vi "3Danalysis240909 cropcalibration with real-time waveforms.vi"() -> ()   [LabVIEW 2024]
uses:
  <vilib>/Utility/file.llb/Read Delimited Spreadsheet (DBL).vi
  <vilib>/Utility/file.llb/Read Delimited Spreadsheet (string).vi
  Global variables/filepath global variable.vi
  Global variables/global for picoscope.vi
  <vilib>/Utility/file.llb/Write Delimited Spreadsheet (DBL).vi
  <vilib>/Utility/file.llb/Write Delimited Spreadsheet (I64).vi
panel:
  in  "round-trip":bool
  in  "fit results":bool
  in  "correction":T1={"vibration removal"=FALSE, "x correct fast/slow"=TRUE, "y correct fast/slow"=TRUE, "z correct fast/slow"=TRUE}
  out "max ch2":u16
  out "max ch1":u16=17224
  out "volume rate [Hz]":dbl=450.6612227351971
  in  "batch":bool
  out "config":bool
  in  "save config":bool
  in  "init frame ofst ch1":dbl
  out "path":path
  out "z ofst":dbl
  in  "auto z adjust":T2={"margin"=100.0, "auto z adj"=FALSE, "average"=10, "use given ofst"=FALSE, "given ofst"=0}
  in  "save file":enum16{"3DU16", "avi", "avia.tif", "none"}(ring)=enum."avia.tif"
  in  "init volume":i64 min=-1 max=9995
  out "Numeric":i32
  out "x-y":dbl=0.003430600045248866
  in  "vol ofst for filesave":i32
  out "x-y 2":dbl=154.19183529983275
  out "x-y 3":dbl=0.0007527999114245176
  in  "save all":bool=TRUE
  out "Array":u16[](array[numeric])=[1044]
  out "Array 2":u16[](array[numeric])
  out "Waveform Graph 8":u16[](graph)=[1044]
  out "Waveform Graph 7":u16[](graph)
  out "Waveform Graph 3":u16[](graph)
  in  "# of vols to save":u32=9 max=9996
  in  "init frame ofst ch2":dbl
  in  "calib using picoscope":bool
  out "error out 2":errorcluster
  out "cal":bool=TRUE
  out "static cropcalib ch2":dbl[][][](array[numeric])
  out "static cropcalib ch1":dbl[][][](array[numeric])=[[[-0.0012324508841086526, -13.277704725109043, 0.9825265622945943, 0.013882930010711092], [-9.275883597421803, 40.97187002025559, 0.26309128953548033, 0.01695088157165565]], [[-0.0037120993202699767, 133.57085155510373, 0.31941814051590384, 0.021131841125054136], [-9.390393874751965, 181.5531741318331, -0.10717785095280981, 0.018933425267278654]], [[0.0019777746813413695, 278.58470887012226, 0.12331601194921626, 0.017358112403776993], [-9.300617403370904, 321.6599217146224, -0.408166255458373, 0.007869360209962234]], [[0.003878363727042984, 422.57664944690487, 0.012423017399425418, 0.008011499786472465], [-9.810808384161477, 461.18609374492786, -0.022657621769615152, 0.006436963821634987]], [[-0.005737681625292825, 565.5516858154322, 0.2650733563737, 0.011263202764196095], [-9.832152645016635, 600.6762263679414, -0.30527039372187453, 0.010318730252671056]], [[8.042249450854295e-07, 707.5829139794733, -0.1207414064195435, 0.0023412830187913803], [-9.87910924649735, 739.8216036823347, 0.005640673976347694, -0.0005605768217188439]], [[-0.01334711027106098, 848.5600859130332, 0.12422403037488547, 0.002919715456556465], [-9.442660667127637, 878.9222143445218, 0.2884952700379346, -0.0006542554942195691]], [[0.0, 990.0108512212238, 0.0, 0.0], [-9.33364564551871, 1018.373465441547, 0.10671859828055268, -0.0003399303862730855]], [[0.0, 1130.6258231987185, 0.0, 0.0], [-9.580976920588036, 1157.4289207081854, -0.046484964058340905, -0.0023746044096836305]], [[0.19067519003123512, 1271.6329414805725, 0.28218230543582085, -0.004007953579247134], [-9.478759959162836, 1296.7982093928567, 0.06815273675590765, -0.005249059904662809]], [[0.002910935849795122, 1411.5924221171872, 0.23076489126866379, -0.0035025104155532653], [-9.327754021590689, 1436.6481286976045, -0.15077568684339113, 0.002054927352480896]], [[0.0045119752683153375, 1551.6884161105997, 0.9967475870149168, 0.005783955565654333], [-9.342246137492738, 1576.5099590441323, -0.036967108722480435, -0.0015882138039450067]], [[0.0012251998944222717, 1691.7091671736623, 0.8828208157286062, 0.004890461811581429], [-8.991691053184148, 1717.2464623070055, 0.42353732985143466, 0.008074427179974693]], [[0.04480350158940928, 1831.6789885716557, 0.2702553130960064, 0.008058123936945851], [-9.520266895758336, 1858.7924624587888, 0.13922336686163864, 0.012889168242776554]], [[0.006579691004563718, 1972.5865362020297, -0.31771324719759314, 0.011874761201387155], [-9.693713496805085, 2000.6691119313275, 0.28434979045685604, 0.006521998044205342]], [[-0.00011619691447528437, 2113.575841906626, 0.027477117752841233, 0.008658919164037509], [-8.4059148140794, 2144.426688166775, -0.0013392330480600891, 0.0034757601889036393]]]
  out "ref image":u16[][](graph)
  out "merged 2":picture
  in  "first calib?":bool
  in  "calib folder":path=path "E:/20241013-235052zebrafish-cropbulkcalib"
  in  "man x correct":dbl[](array[numeric])=[0.0, 0.0, 0.0, 0.0, 0.0, 0.0, 0.0, 0.0, 0.0, 0.0, 0.0, 0.0, 0.0, 0.0, 0.0, 0.0] format="%_3g"
  out "xcutcalib":bool
  in  "save xcutcalib":bool
  out "Waveform Graph 6":dbl[][](graph)
  in  "add xcutcalib":bool
  out "Waveform Graph 5":dbl[][](graph)=[[71.24917145755833, 2.611229946524065], [52.12883880825057, 96.52276455026455], [38.370065789473685, 37.02559300873908], [109.29258898776419, 117.5164798671648], [109.03552721356218, 113.07896244046542], [107.5345264511574, 111.91266505636071], [101.79099323375462, 108.80995217599235], [81.80626577898215, 91.38536842105262], [76.35199183363878, 81.89281794462502], [72.85646288715512, 77.08998393172541], [70.33839267741641, 73.63359060670481], [68.91633042357225, 71.23733432369326], [68.61642295097899, 70.59161782206286], [67.06026334942868, 69.3341155147388], [67.74688487608418, 68.88457267871622], [67.23388367805843, 67.52512049939843]]
  out "Waveform Graph 4":dbl[][](graph)=[[70.75082854244167, 12.808059587471355, 2.629934210526315, 14.534830367074527, 16.427308035479975, 17.7857922739422, 22.1671837099451, 9.975237111191262, 9.040092700463049, 10.394476704747461, 12.436049890733301, 13.007639351673383, 13.537171153329393, 13.652122809925942, 13.660225864725732, 13.787552156319304], [2.611229946524065, 2.787949735449729, 2.7521847690387027, 14.601328352013269, 18.22516127087478, 18.055853462157813, 21.7295600191296, 12.989368421052625, 8.892359420239849, 10.20478995530609, 12.280460403088203, 13.044423160691835, 13.582757039632213, 13.732063344670266, 13.630206965107035, 13.843818558527587]]
  out "calib errors":dbl[][](graph)=[[71.24917145755833, 52.12883880825057, 38.370065789473685, 109.29258898776419, 109.03552721356218, 107.5345264511574, 101.79099323375462, 81.80626577898215, 76.35199183363878, 72.85646288715512, 70.33839267741641, 68.91633042357225, 68.61642295097899, 67.06026334942868, 67.74688487608418, 67.23388367805843], [2.611229946524065, 96.52276455026455, 37.02559300873908, 117.5164798671648, 113.07896244046542, 111.91266505636071, 108.80995217599235, 91.38536842105262, 81.89281794462502, 77.08998393172541, 73.63359060670481, 71.23733432369326, 70.59161782206286, 69.3341155147388, 68.88457267871622, 67.52512049939843]]
  out "Waveform Graph 2":u64[][](graph)
  out "mag corr ch2":dbl=0.9999999999999987
  out "size(s) 2":i32[](array[numeric])=[344, 346]
  out "#ofvoxels":i32[](array[numeric])=[2, 144, 2304]
  in  "y shift comp ch2":dbl=2.0 format="%_4g"
  out "# of slices per frame":dbl=16.0
  out "coeffs ch2":T3={"coeffs for r adjust"=[519.0152004188965, 310.5655915232708, 70.01299823861439, 7.02374490371761, 0.263935632321602], "coeffs for x pos adjust"=[1129.1985384616178, -0.06820417207386949, 3.261911031170097e-08, -3.700712469960341e-12, -2.2526696193466402e-15, 2.275859361243603e-19, 4.209771129915532e-23, -5.09041527821271e-27, -4.152675622145259e-31, 5.315442386029638e-35, 2.2654166541347624e-39, -2.8567558128164638e-43, -6.398399651393965e-48, 7.62901113711002e-52, 7.223314072712311e-57, -8.008405878791859e-61], "coeffs for intensity adjust"=[0.058988135271943375, -6.250993723417386e-05, 8.465587569932774e-07, -2.944632303001578e-09, 4.603084712096755e-12, -3.778602476142126e-15, 1.6979803184001706e-18, -3.9600508630542766e-22, 3.7530066428820694e-26]}
  out "coeffs ch1":T3={"coeffs for r adjust"=[17.10761405696684, 7.84114849852129, 1.7677363155338985, 0.2069198771701287, 0.00932990152601304], "coeffs for x pos adjust"=[1127.3789093477487, -0.06827960368149495, 3.2476822001437325e-08, 1.2710261197144785e-13, -1.3608202177260485e-15, 1.4043859987815547e-21, 2.104622239338711e-23, 2.30596280455575e-28, -2.3225210012230083e-31, -9.089899485608927e-36, 2.1092005655095755e-39, 9.893885524186623e-44, -1.2826034157079897e-47, -4.393969803780215e-52, 4.214036083794186e-56, 6.97605374735289e-61, -5.591200085114606e-65], "coeffs for intensity adjust"=[0.25889415470638116, -0.00016368169857389878, 1.1910443462708163e-08, -7.647385084110969e-10, 1.8842781690841883e-12, -1.906465046959414e-15, 9.982378310740631e-19, -2.6840743111736396e-22, 2.938746954924419e-26]}
  out "img scan voltage":dbl[][](array[numeric])
  out "img scan tangent":dbl[][](array[numeric])
  out "calib index":i32
  out "Waveform Graph":u32[][](graph)=[[15301, 15180, 15264, 15156, 15317, 15620, 15556, 15291, 15455, 15405, 15401, 15373, 15584, 15573, 15767, 15492, 15691, 15604, 15561, 15794, 15664, 15376, 15642, 15407, 15469, 15364, 15405, 15434, 15394, 15413, 15350, 15460, 15316, 15440, 15429, 15553, 15564, 15422, 15390, 15723, 15577, 15625, 15805, 15738, 15559, 15673, 15778, 15951, 15719, 15813, 15643, 15950, 15843, 15867, 15752, 15687, 15565, 15831, 15737, 15690, 15741, 15588, 15471, 15668, 15745, 15718, 15687, 15627, 15417, 15716, 15742, 15760, 15744, 15903, 15757, 15817, 15715, 15772, 15822, 15917, 15764, 15955, 15688, 15823, 15723, 15617, 15641, 15498, 15509, 15540, 15467, 15681, 15463, 15503, 15416, 15393, 15441, 15439, 15466, 15298, 15311, 15441, 15260, 15298, 15258, 15267, 15341, 15224, 15222, 15120, 15226, 15313, 15275, 15176, 15268, 15210, 15155, 15201, 15095, 15249, 15176, 15248, 15220, 15296, 15148, 15124, 15152, 15276, 15240, 15128, 15162, 15171, 15217, 15209, 15238, 15355, 15305, 15141, 15199, 15275, 15223, 15324, 15184, 15222, 15158, 15279, 15288, 15313, 15254, 15159, 15370, 15393, 15448, 15274, 15475, 15438, 15469, 15554, 15779, 15661, 15709, 15811, 15752, 15747, 15674, 15677, 15732, 15441, 15664, 15538, 15479, 15524, 15353, 15443, 15486, 15434, 15412, 15413, 15332, 15417, 15385, 15511, 15304, 15327, 15381, 15325, 15492, 15474, 15428, 15381, 15710, 15723, 15643, 15578, 15595, 15577, 15710, 15546, 15584, 15590, 15497, 15653, 15634, 15476, 15548, 15538, 15617, 15466, 15546, 15575, 15482, 15436, 15510, 15547, 15364, 15570, 15524, 15525, 15401, 15598, 15591, 15501, 15572, 15609, 15540, 15693, 15490, 15453, 15613, 15544, 15603, 15536, 15393, 15609, 15422, 15500, 15552, 15330, 15306, 15418, 15271, 15374, 15347, 15270, 15334, 15281, 15261, 15290, 15296, 15137, 15348, 15212, 15159, 15360, 15150, 15233, 15106, 15189, 15153, 15232, 15155, 15364, 15279, 15248, 15187, 15153, 15122, 15164, 15379, 15274, 15347, 15249, 15096, 15359, 15362, 15224, 15313, 15428, 15264, 15307, 15212, 15090, 15264, 15277, 15291, 15138, 15253, 15329, 15351, 15295, 15246, 15360, 15238, 15463, 15316, 15448, 15364, 15595, 15507, 15632, 15755, 16022, 16075, 16206, 16022, 16142, 16221, 16087, 15909, 15837, 15636, 15936, 15910, 15764, 15799, 15649, 15868, 15776, 15651, 15764, 15618, 15379, 15599, 15447, 15560, 15468, 15370, 15563, 15391, 15358, 15343, 15440, 15501, 15404, 15597, 15488, 15308, 15516, 15654, 15472, 15411, 15486, 15716, 15512, 15710, 15658, 15524, 15441, 15730, 15407, 15472, 15352, 15539, 15410, 15505, 15504, 15409, 15402, 15634, 15370, 15422, 15453, 15528, 15406, 15400, 15524, 15386, 15511, 15444, 15512, 15377, 15500, 15715, 15412, 15544, 15388, 15328, 15393, 15459, 15265, 15314, 15280, 15236, 15370, 15422, 15418, 15205, 15193, 15347, 15173, 15370, 15242, 15228, 15060, 15265, 15166, 15148, 15284, 15223, 15229, 15300, 15278, 15142, 15058, 15158, 15119, 15289, 15124, 15233, 15118, 15208, 15111, 15234, 15133, 15042, 15094, 15042, 15032, 15002, 15002, 14881, 14742, 14852, 14737, 14936, 14673, 14649, 14760, 14733, 14748, 14659, 14623, 14658, 14696, 14688, 14762, 14665, 14769, 14866, 14937, 15108, 14998, 15277, 15463, 15587, 15444, 15777, 15716, 15491, 15710, 15500, 15671, 15793, 15788, 15636, 15796, 15739, 15537, 15236, 15566, 15438, 15293, 15155, 15182, 15237, 15280, 15128, 15231, 14931, 15277, 14907, 14833, 14939, 14989, 14857, 14833, 14881, 14717, 14877, 14883, 14851, 14867, 14821, 14647, 14814, 14897, 14835, 14793, 14950, 14956, 14795, 14876, 14850, 14888, 14865, 14696, 14836, 14783, 14891, 14790, 14911, 14817, 14898, 14793, 14971, 14870, 14925, 14735, 14810, 14636, 14845, 14818, 14698, 14750, 14783, 14724, 14762, 14697, 14790, 14881, 14914, 14826, 14649, 14710, 14946, 14827, 14735, 14720, 14626, 14787, 14673, 14606, 14648, 14823, 14654, 14549, 14721, 14744, 14830, 14769, 14608, 14568, 14724, 14723, 14668, 14814, 14601, 14710, 14865, 14640, 14657, 14722, 14646, 14625, 14607, 14694, 14631, 14864, 14665, 14746, 14790, 14679, 14656, 14511, 14679, 14547, 14610, 14816, 14836, 14622, 14726, 15028, 14747, 14699, 14809, 14849, 14934, 14798, 15011, 14970, 14942, 14926, 15361, 15383, 15318, 15654, 15568, 15877, 15922, 16129, 16325, 16195, 16142, 16324, 15970, 16153, 16258, 16122, 16121, 15864, 15996, 15776, 15984, 15895, 15770, 15641, 15841, 15542, 15614, 15569, 15408, 15432, 15397, 15399, 15281, 15335, 15037, 15085, 14974, 15158, 15012, 14836, 15038, 14777, 14954, 14924, 14903, 14761, 14934, 14849, 14847, 14636, 14963, 14896, 14905, 14930, 15016, 14904, 14889, 14977, 14884, 14887, 14727, 14785, 14783, 14768, 14720, 14690, 14917, 14744, 14840, 14804, 14766, 14829, 14834, 14711, 14745, 14869, 14833, 14779, 14742, 14837, 14866, 14951, 14722, 14784, 14727, 14825, 14674, 14801, 14805, 14658, 14887, 14875, 14775, 14606, 14616, 14529, 14680, 14740, 14578, 14672, 14813, 14756, 14670, 14693, 14612, 14793, 14597, 14734, 14679, 14724, 14685, 14677, 14654, 14655, 14678, 14675, 14513, 14571, 14668, 14665, 14616, 14624, 14663, 14614, 14754, 14637, 14634, 14619, 14753, 14686, 14505, 14700, 14550, 14684, 14589, 14762, 14776, 14836, 14635, 14801, 15007, 15117, 15100, 15439, 15491, 15771, 15906, 16022, 16368, 16512, 16330, 16351, 16557, 16465, 16406, 16234, 16591, 16446, 16480, 16250, 16315, 16147, 16060, 16079, 16094, 15904, 15863, 15932, 15882, 15891, 15683, 15596, 15649, 15525, 15478, 15666, 15460, 15409, 15276, 15227, 15141, 15230, 15059, 15197, 14980, 14852, 14745, 14895, 14902, 14975, 14783, 14747, 14806, 14615, 14725, 14654, 14869, 14645, 14679, 14727, 14569, 14636, 14908, 14606, 14674, 14774, 14843, 14803, 14841, 14843, 14818, 14781, 14918, 14820, 14756, 14862, 14753, 14709, 14728, 14766, 14850, 14664, 14686, 14748, 14838, 14594, 14634, 14706, 14604, 14633, 14584, 14693, 14670, 14469, 14631, 14633, 14634, 14639, 14533, 14704, 14649, 14757, 14567, 14679, 14508, 14521, 14695, 14630, 14850, 14637, 14665, 14690, 14741, 14705, 14606, 14787, 14585, 14653, 14552, 14709, 14690, 14607, 14611, 14761, 14773, 14690, 14538, 14702, 14738, 14767, 14710, 14460, 14620, 14837, 14753, 14661, 14781, 14701, 14799, 14908, 14827, 15123, 15229, 15246, 15510, 15604, 15760, 16237, 16402, 16499, 16640, 16630, 16865, 16713, 16772, 16986, 17048, 16820, 17014, 17012, 16803, 16863, 16755, 16959, 16780, 16746, 16827, 16793, 16578, 16902, 16565, 16658, 16675, 16497, 16458, 16430, 16427, 16376, 16348, 16316, 16314, 16299, 16308, 16615, 16241, 16331, 16279, 16335, 16241, 15910, 15826, 15634, 15615, 15284, 15254, 15096, 14971, 14700, 14734, 14773, 14798, 14644, 14652, 14671, 14674, 14664, 14511, 14692, 14763, 14704, 14759, 14553, 14655, 14653, 14709, 14624, 14626, 14798, 14717, 14682, 14534, 14682, 14583, 14548, 14461, 14605, 14458, 14579, 14654, 14660, 14631, 14606, 14737, 14701, 14810, 14597, 14712, 14469, 14742, 14784, 14763, 14537, 14784, 14711, 14880, 14778, 14801, 14789, 14826, 14816, 14795, 14786, 15015, 14997, 14956, 15024, 14709, 14923, 14843, 15055, 15216, 14971, 15234, 15172, 14933, 15048, 15215, 14970, 15048, 14963, 15170, 15194, 15187, 14911, 14855, 15080, 15189, 15258, 15303, 15139, 15331, 15551, 15836, 15861, 15969, 16312, 16430, 16568, 16676, 17392, 17468, 17768, 17693, 17963, 18003, 17922, 18241, 18356, 18506, 18505, 18693, 18834, 18522, 18645, 18971, 18831, 19145, 19262, 19202, 19282, 19163, 19920, 19966, 20063, 20348, 20393, 20656, 20340, 21145, 21549, 21592, 22895, 23897, 24817, 26484, 27677, 28989, 30335, 31522, 32712, 33150, 33951, 34337, 33384, 33011, 31426, 29622, 27294, 25484, 23051, 20348, 19043, 17525, 16719, 16071, 15893, 15557, 15642, 15478, 15709, 15737, 15436, 15783, 15635, 15433, 15632, 15632, 15509, 15537, 15450, 15605, 15399, 15681, 15592, 15674, 15625, 15525, 15509, 15757, 15625, 15765, 15896, 16007, 15916, 15913, 15957, 15909, 16022, 15915, 16044, 15928, 16205, 16212, 15998, 16200, 15978, 16027, 16055, 16251, 16221, 15986, 15900, 16181, 16011, 16126, 16144, 16104, 15950, 16110, 16250, 16178, 15817, 15999, 15876, 15970, 15988, 16103, 16080, 16090, 16142, 16097, 15951, 16043, 16001, 16185, 16033, 16197, 16194, 16187, 16293, 16448, 16389, 16439, 16771, 16725, 17242, 17347, 17859, 18357, 18497, 19124, 18931, 19384, 19557, 19681, 20120, 20401, 20902, 20890, 21244, 21383, 21631, 21445, 21859, 21581, 22396, 22624, 22629, 22872, 23615, 23902, 24218, 24837, 25984, 27149, 28740, 29966, 31555, 33231, 34755, 35668, 37514, 41116, 44002, 48952, 53923, 60849, 67906, 75888, 84944, 92910, 100381, 107495, 114716, 119015, 121334, 123649, 124437, 120797, 114049, 105794, 96821, 84687, 70486, 58082, 44862, 35256, 27393, 22565, 19113, 17558, 16721, 16534, 16333, 16339, 16347, 16226, 16349, 16177, 16227, 16152, 16088, 16127, 16170, 16022, 16206, 16060, 15819, 15950, 16096, 15893, 16030, 15980, 15961, 15897, 15997, 16092, 15901, 16154, 16074, 16032, 16079, 15908, 15981, 15858, 15948, 15991, 15950, 15907, 15791, 15741, 15870, 15941, 15946, 15786, 15735, 15883, 15833, 15812, 15917, 15778, 15816, 15824, 15904, 16092, 15925, 15850, 15892, 15870, 16134, 16127, 15951, 15940, 16044, 15942, 15967, 16154, 16178, 16250, 16305, 16374, 16485, 16677, 17020, 17399, 17653, 18134, 18430, 18725, 19268, 19703, 20036, 20607, 20881, 21617, 21808, 22208, 22703, 23272, 23742, 24224, 25206, 25741, 26436, 26115, 26837, 27022, 27879, 28914, 29039, 30172, 31220, 32066, 33038, 33999, 35051, 35854, 37878, 40694, 44209, 48835, 53423, 59090, 66638, 73627, 84244, 93544, 107457, 122595, 140161, 158551, 176805, 195989, 216903, 237255, 253503, 268650, 279752, 288924, 294235, 297628, 296038, 287332, 278665, 263556, 243244, 221305, 195837, 166539, 136516, 105426, 75906, 53503, 39346, 29244, 22700, 19333, 18204, 17399, 17089, 17127, 16970, 16678, 16734, 16750, 16657, 16567, 16785, 16628, 16332, 16398, 16470, 16429, 16394, 16557, 16197, 16424, 16217, 16243, 16481, 16269, 16480, 16195, 16094, 16229, 16129, 16155, 16125, 16097, 16103, 15991, 16154, 15764, 16125, 16167, 16082, 16010, 15905, 16131, 15931, 16049, 16092, 16023, 16103, 16091, 16012, 16082, 15955, 16083, 16025, 16045, 15977, 16060, 16144, 16213, 16027, 16082, 16235, 16311, 16377, 16503, 16775, 16862, 17475, 17701, 18469, 18731, 19442, 19969, 20370, 21112, 21671, 22136, 23022, 23572, 24091, 24722, 25933, 26396, 26817, 27431, 28425, 29086, 29942, 30624, 31583, 33102, 34332, 35298, 36413, 37376, 38747, 39967, 43311, 47174, 49971, 54701, 57287, 59902, 63295, 66811, 71971, 78251, 87577, 99880, 113736, 131859, 153016, 178039, 206189, 239140, 268322, 301593, 333225, 367689, 398869, 428520, 451155, 475148, 489399, 497230, 503148, 496024, 486052, 473743, 459727, 440198, 423502, 401541, 378537, 350159, 317117, 283508, 249811, 212312, 172174, 130532, 93652, 63983, 45225, 34266, 26456, 22357, 19836, 18750, 18252, 17894, 17777, 17481, 17485, 17554, 17437, 17303, 17283, 17111, 17217, 17206, 17221, 17107, 17105, 16961, 16998, 16806, 16832, 16863, 16808, 16803, 16745, 16679, 16747, 16551, 16469, 16574, 16435, 16529, 16401, 16521, 16386, 16392, 16523, 16342, 16525, 16259, 16297, 16355, 16263, 16338, 16314, 16273, 16224, 16130, 16484, 16470, 16374, 16335, 16439, 16365, 16735, 16643, 16905, 17006, 17275, 17985, 18159, 19047, 19437, 20108, 20875, 21610, 22120, 22948, 24140, 24131, 25489, 26193, 26968, 28297, 29738, 30483, 31666, 32227, 33636, 34398, 34059, 35223, 36490, 36884, 38504, 40271, 41945, 44509, 47280, 48477, 51090, 54262, 56936, 61006, 66133, 71868, 79670, 88305, 99993, 111659, 128041, 143678, 164564, 188426, 212219, 243102, 279213, 317533, 361157, 407173, 451353, 496387, 540920, 589454, 628126, 669232, 700813, 723519, 745001, 753018, 752391, 740749, 723123, 691046, 658326, 620040, 572513, 527741, 480657, 444358, 410016, 378605, 350538, 322320, 291428, 258834, 225020, 189363, 152976, 118813, 86963, 61562, 44560, 34493, 27353, 24224, 21579, 19913, 19389, 19236, 18812, 18744, 18724, 18475, 18422, 18363, 18216, 18115, 17977, 17841, 17896, 18034, 17844, 18199, 17500, 17515, 17515, 17496, 17497, 17255, 17290, 17574, 17424, 17177, 17375, 17090, 17144, 17219, 17022, 17080, 17145, 16820, 17223, 17039, 17189, 16899, 17020, 16870, 16910, 16866, 17041, 16979, 16909, 17002, 16944, 17150, 17566, 17899, 18236, 18515, 19087, 19838, 20625, 21161, 22236, 23021, 23997, 24730, 25887, 27082, 27799, 28365, 29108, 30249, 31803, 32735, 33182, 34289, 35800, 37800, 38796, 40330, 41050, 42229, 44197, 45186, 46340, 47995, 51153, 53820, 57457, 60830, 66370, 70884, 76806, 82883, 88504, 96097, 106036, 119146, 135853, 159213, 184956, 218869, 257150, 303167, 351380, 404496, 461094, 516175, 572027, 633124, 688319, 738230, 787014, 827991, 854865, 881463, 896306, 910597, 913862, 913067, 906683, 890807, 865170, 831071, 795584, 754028, 709973, 662118, 605784, 549409, 483865, 419856, 360697, 315672, 280400, 253947, 234130, 214854, 194686, 173041, 149605, 127645, 104234, 84306, 65189, 51366, 39446, 32019, 26412, 23264, 21272, 20159, 19385, 18610, 18414, 18093, 18490, 17971, 17983, 17783, 17851, 17674, 17628, 17318, 17252, 17442, 17439, 17331, 17261, 17127, 17244, 16886, 16953, 16784, 16641, 16852, 16628, 16669, 16711, 16434, 16638, 16463, 16581, 16567, 16486, 16240, 16433, 16524, 16551, 16194, 16391, 16314, 16489, 16680, 17180, 17175, 17711, 18422, 19049, 19979, 21200, 21935, 22972, 23556, 25590, 26261, 27006, 28339, 28906, 30104, 30911, 32480, 33461, 35388, 36464, 37352, 38800, 40399, 41320, 42713, 45053, 47280, 49848, 52384, 54499, 58600, 60782, 63994, 67586, 69716, 74103, 77534, 84424, 91208, 99851, 110435, 124005, 137527, 155612, 178442, 202188, 235450, 273699, 319248, 372231, 433490, 501830, 576537, 653111, 732092, 812185, 889041, 962405, 1033476, 1096394, 1142818, 1173475, 1192354, 1200630, 1192201, 1172933, 1139546, 1089841, 1040146, 986591, 927992, 870181, 806735, 746934, 685563, 632047, 584453, 533421, 482557, 433064, 381002, 323084, 266939, 216421, 175486, 147291, 125611, 112236, 104304, 94351, 85259, 75673, 66289, 57941, 50597, 43241, 38954, 33458, 29350, 25379, 23511, 21532, 20226, 19809, 18965, 18703, 18501, 18209, 18260, 18141, 17817, 17809, 18016, 17674, 17697, 17429, 17443, 17414, 17227, 17312, 17028, 17105, 17088, 17094, 17016, 16913, 16813, 16998, 16852, 16557, 16827, 16800, 16751, 16651, 16644, 16786, 16902, 17043, 17034, 17564, 17724, 18440, 19136, 19888, 20738, 21984, 23073, 24714, 25388, 26621, 28099, 29669, 30688, 32055, 32735, 34008, 35241, 35868, 37543, 38391, 39021, 40822, 42295, 45423, 45800, 49099, 50955, 52919, 55654, 59539, 62706, 67003, 70922, 76452, 82783, 89017, 95961, 102930, 111409, 118810, 128557, 140490, 154271, 170561, 192744, 221950, 258542, 301489, 352767, 409571, 475568, 546229, 620262, 699762, 783523, 874514, 959011, 1044943, 1120847, 1187540, 1248777, 1293721, 1333230, 1359942, 1379028, 1382262, 1379460, 1359103, 1327999, 1285059, 1231617, 1164257, 1091238, 1007154, 928419, 844405, 757878, 676229, 597066, 528033, 463441, 413333, 374781, 335717, 300607, 263367, 229745, 193155, 160808, 128937, 102926, 82811, 67352, 56486, 49754, 45587, 42542, 40256, 38294, 35989, 34950, 33131, 31780, 29795, 27955, 26516, 24316, 22921, 21806, 20404, 19737, 19399, 19001, 18452, 18706, 18467, 18304, 18158, 18056, 17919, 17801, 18174, 17694, 17760, 17705, 17767, 17437, 17521, 17338, 17410, 17443, 17280, 17343, 17149, 17543, 17318, 17788, 17827, 17840, 18200, 18793, 19208, 19827, 20694, 21466, 22573, 23700, 24945, 25659, 27197, 29110, 29533, 31317, 32834, 34114, 34715, 36219, 38039, 38475, 39989, 41731, 43043, 44588, 45833, 47268, 48769, 49436, 51832, 54445, 57775, 59840, 63742, 67764, 70830, 75375, 81209, 87777, 93275, 103706, 112868, 125799, 137302, 156220, 175226, 197889, 226567, 257984, 297377, 341021, 390206, 450937, 522808, 601241, 691414, 781338, 882139, 984069, 1085111, 1187802, 1288509, 1381524, 1463138, 1534083, 1585526, 1617605, 1633580, 1624674, 1600301, 1560683, 1505553, 1441754, 1362876, 1288571, 1214588, 1136801, 1063451, 994504, 918425, 842202, 764751, 681209, 603591, 530105, 463057, 397166, 338045, 287495, 243163, 208503, 181413, 163218, 144555, 128059, 114225, 99374, 87439, 75751, 67156, 57580, 50017, 43598, 38676, 34192, 31828, 30513, 29648, 28873, 28263, 27857, 27605, 26534, 26224, 25603, 24809, 22981, 22510, 21546, 20835, 19857, 19264, 19073, 18890, 18430, 18477, 18180, 18055, 18322, 17982, 17782, 17589, 17392, 17555, 17257, 17398, 17054, 16987, 16721, 16538, 16379, 16262, 15924, 15643, 15674, 15358, 15222, 15328, 15019, 14994, 15002, 15053, 14869, 14782, 14709, 14755, 14624, 14632, 14699, 14720, 14786, 14800, 14606, 14729, 14808, 14642, 14714, 14677, 14568, 14415, 14610, 14635, 14451, 14498, 14499, 14383, 14464, 14469, 14470, 14537, 14432, 14429, 14424, 14405]]
  in  "init vol":i32
  in  "skip":i32=30 min=1
  out "coeffs":bool
  out "error out":errorcluster
  out "config cluster":T4={"xy cut pos correct"=[[0.0, 0.0], [0.0, 0.0], [0.0, 0.0], [0.0, 0.0], [0.0, 0.0], [0.0, 0.0], [0.0, 0.0], [0.0, 0.0], [0.0, 0.0], [0.0, 0.0], [0.0, 0.0], [0.0, 0.0], [0.0, 0.0], [0.0, 0.0], [0.0, 0.0], [0.0, 0.0]], "3D reconst config"={"xyz pos"=[68, 22, 14], "color 4"={"color array"=[0, 8388736, 16711680, 16776960, 16776960, 16711680, 16448250, 16448250], "num of colors"=4, "max"=7000.900000000023, "min"=100.0}, "autogain"=TRUE, "zoom"=1.0, "slice(T)/stack(F)"=FALSE, "xy cut mag"=0.999999999999986, "xy cut ofst"=0.0, "z/xy comp"=1.0, "y shift comp"=0.0, "max plot"=TRUE, "oblique angle [deg]"=0.0, "voxel size z [um]"=2.47291183688844, "voxel size xy[um]"=0.4095, "reverse v"=FALSE, "reverse h"=TRUE, "3D reconstruction"=TRUE, "reverse z"=FALSE}, "xy cut pos"=[[0.0, 0.0], [0.0, 0.0], [0.0, 0.0], [0.0, 0.0], [0.0, 0.0], [0.0, 0.0], [0.0, 0.0], [0.0, 0.0], [0.0, 0.0], [0.0, 0.0], [0.0, 0.0], [0.0, 0.0], [0.0, 0.0], [0.0, 0.0], [0.0, 0.0], [0.0, 0.0]], "AOD scan speed ratio"=7.0, "Nx"=142.71428571, "stack method"=enum."0pad to x", "y shift"=-3}
  out "voxel number":i32[](array[numeric])=[32, 141, 143]
  in  "Zoom 2":sgl=1.9000002 format="%_3g"
  in  "Cluster 2":T5={"colors 2"=[{"color array"=[0, 16711680, 16776960, 16448250, 16776960, 16711680, 16448250, 16448250], "num of colors"=4, "max"=20300.0, "min"=100.0}, {"color array"=[0, 65280, 16711680, 16448250, 16776960, 16711680, 16448250, 16448250], "num of colors"=2, "max"=400.0, "min"=140.0}, {"color array"=[0, 16711680, 16448250, 16448250, 16776960, 16711680, 16448250, 16448250], "num of colors"=2, "max"=12500.0, "min"=0.0}, {"color array"=[0, 255, 16448250, 16448250, 16776960, 16711680, 16448250, 16448250], "num of colors"=2, "max"=1.01, "min"=0.0}, {"color array"=[0, 65280, 16448250, 16448250, 16776960, 16711680, 16448250, 16448250], "num of colors"=3, "max"=1.0, "min"=0.0}, {"color array"=[0, 255, 16448250, 16448250, 16776960, 16711680, 16448250, 16448250], "num of colors"=2, "max"=1.0099999999999991, "min"=0.0}], "on/off 2"=[TRUE, TRUE, FALSE, FALSE, FALSE, FALSE], "fast/slow"=TRUE, "on/off"=TRUE} {"colors 2"."min" step=0.01 format="%_2f"; "colors 2"."max" step=0.1 format="%_3f"}
  out "voxel size":dbl[](array[numeric])=[2.47291183688844, 0.4095, 0.4095]
  in  "stack method":T6(ring)=enum."0pad to x"
  out "# of volumes":dbl=2500.0
  out "roop time":dbl=0.7064968999984558
  in  "most recent":bool
  in  "folderpath":path=path "E:/20241013-235254zebrafish"
  out "timestamp":dbl[](array[numeric]) format="%#_12g"
  out "int frame ch2":dbl
  out "int frame ch1":dbl
  out "bytes per frame":i64=663560
  out "frames per vol":dbl=2.0
  in  "3D config":T7={"xyz pos"=[68, 22, 14], "color 4"={"color array"=[0, 8388736, 16711680, 16776960, 16776960, 16711680, 16448250, 16448250], "num of colors"=4, "max"=7000.900000000023, "min"=100.0}, "autogain"=TRUE, "zoom"=1.0, "slice(T)/stack(F)"=FALSE, "xy cut mag"=0.999999999999986, "xy cut ofst"=0.0, "z/xy comp"=1.0, "y shift comp"=0.0, "max plot"=TRUE, "oblique angle [deg]"=0.0, "voxel size z [um]"=2.47291183688844, "voxel size xy[um]"=0.4095, "reverse v"=FALSE, "reverse h"=TRUE, "3D reconstruction"=TRUE, "reverse z"=FALSE} {"oblique angle [deg]" format="%_4g"; "y shift comp" format="%_4g"; "z/xy comp" format="%_4g"; "xy cut mag" format="%_4g"; "zoom" format="%_3g"; "color 4"."min" step=0.01 format="%_2f"; "color 4"."max" step=0.1 format="%_3f"}
  in  "mag correct":dbl=0.9999999999999999 format="%_5g"
  in  "2color":bool
  out "basic info":dbl[](array[numeric])=[2.0, 16.0, 142.71428571, 7.0, 1105.2, 10.0]
  in  "page":i32
  out "# of frames":dbl=5000.0
  out "frame's init pos in x":dbl[][](array[numeric])=[[0.0, 1835.00901738322], [114.51851696314236, 1721.147101789565], [232.0020802680026, 1603.7715933557456], [348.14555636837696, 1489.3931858186936], [462.566358639522, 1375.7385908149276], [579.2325307907199, 1258.8475197694584], [693.9573343258472, 1145.2327344550233], [808.0498359122519, 1031.3113628318458], [924.0289031657775, 915.7950185906724], [1037.9895674693335, 802.6538134765885], [1151.8597552062292, 688.8875445391162], [1266.303305871278, 573.8303042476285], [1379.5189602745013, 460.50349291965074], [1492.7992407967668, 346.3820388319155], [1607.3275809299998, 231.6954939592598], [1721.0230196410016, 118.6551055908842]]
  out "time intervals":dbl[][](graph)
  in  "vol index":i64 min=-1 max=49
  in  "stop":bool
  in  "rel mag ch2":dbl=0.9999999999999988 format="%_5g"
  in  "v shift":i32=-3
  in  "h shift":i32=-9
  out "merged":picture
  out "monitor index":i32=68
  # "1ボリュームあたりのカメラフレーム数\nカメラフレームあたりのXYフレーム数\nXYフレームのＸピクセル数\nratio between AOD & img scan\ng2 period [us]\ndead time for burst [us]"
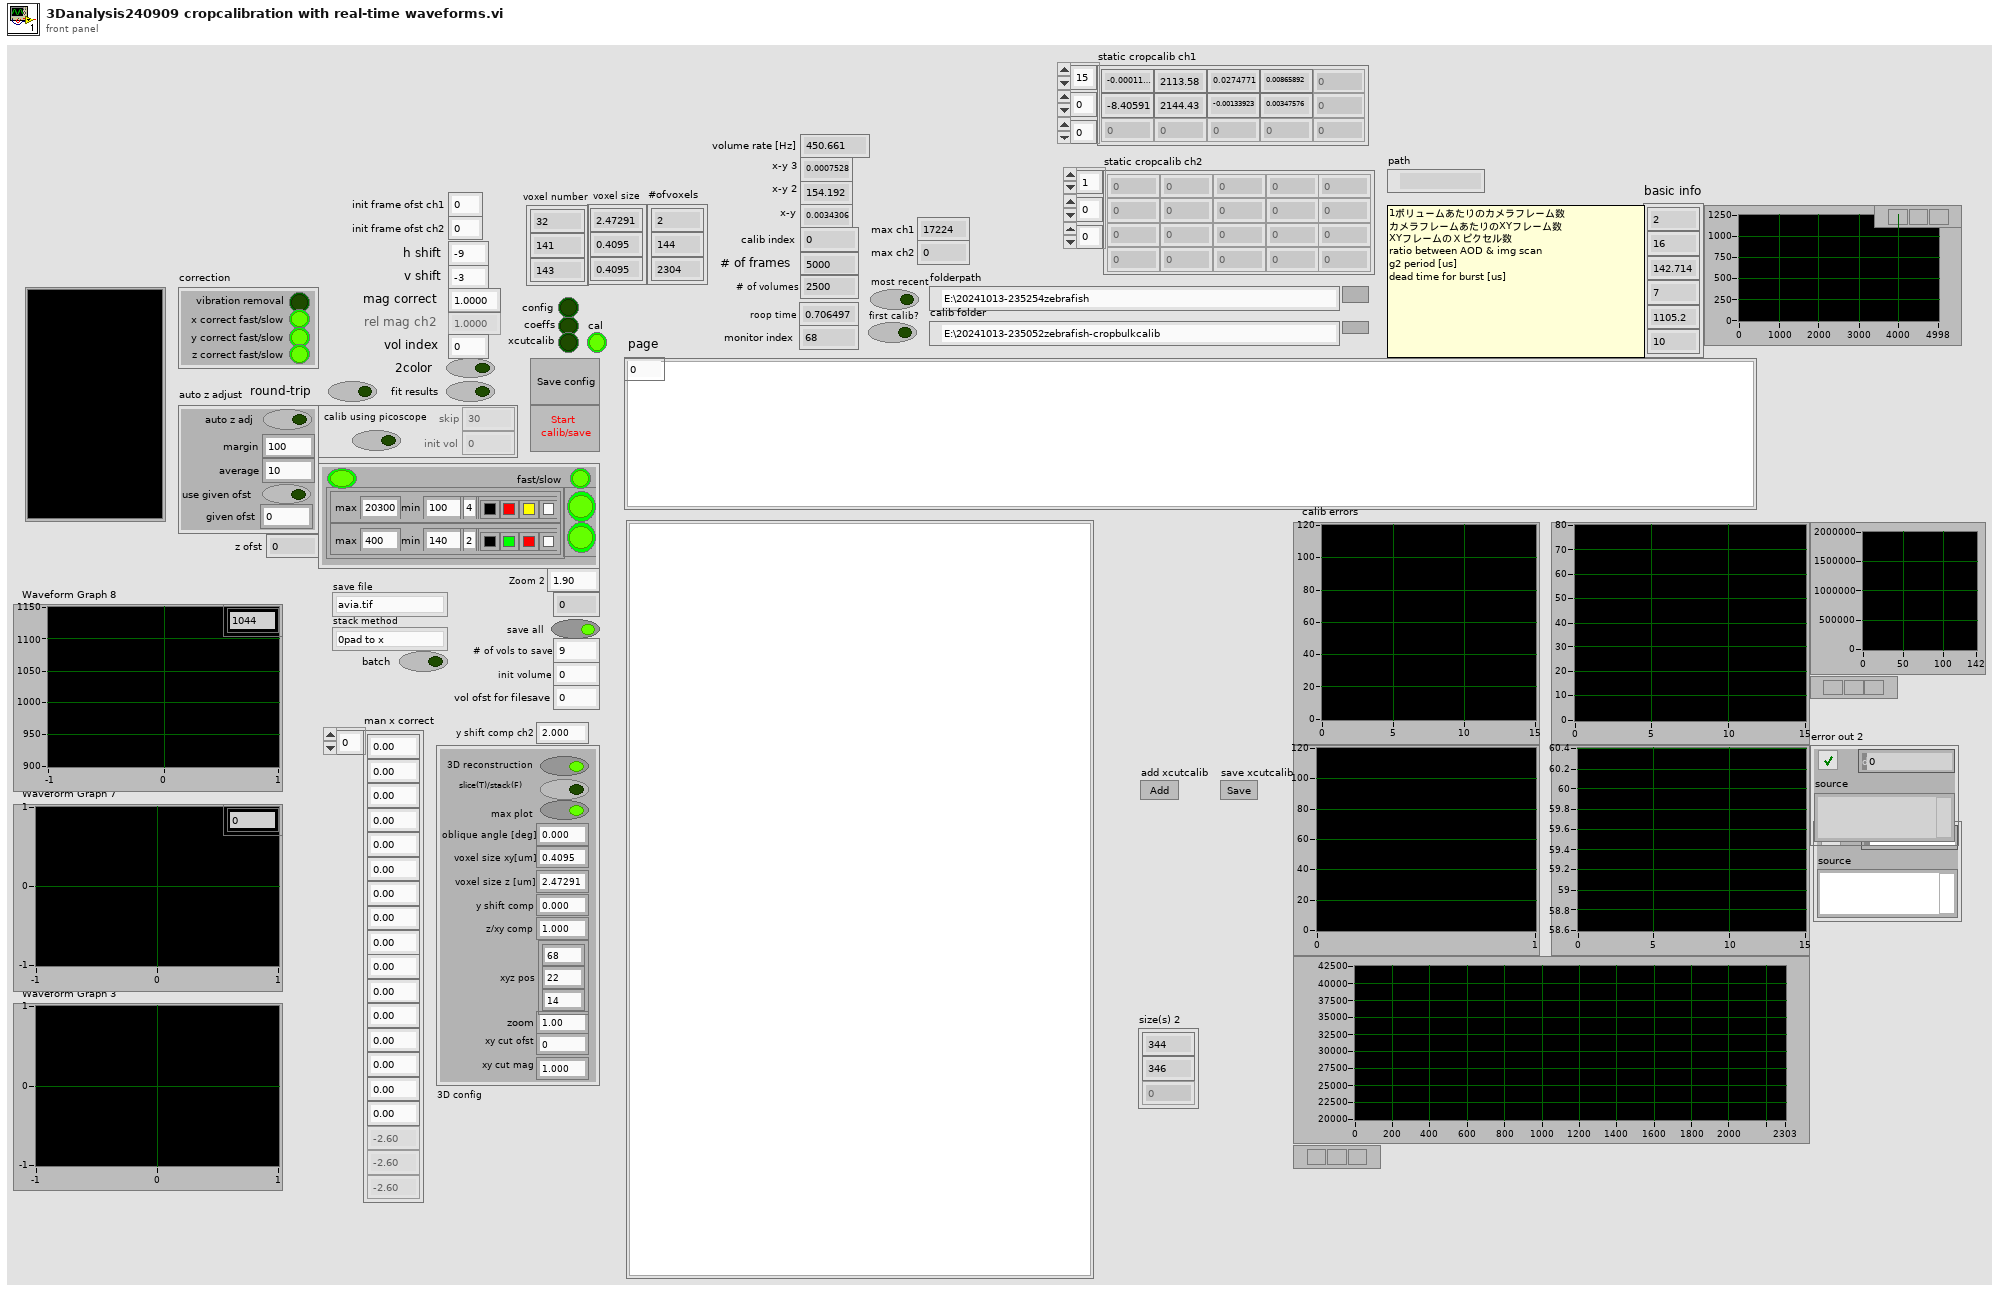
[diagram p1: front panel]
types:
  T1 = cluster{"vibration removal":bool, "x correct fast/slow":bool, "y correct fast/slow":bool, "z correct fast/slow":bool}
  T2 = cluster{"margin":dbl, "auto z adj":bool, "average":i32, "use given ofst":bool, "given ofst":i32}
  T3 = cluster{"coeffs for r adjust":dbl[], "coeffs for x pos adjust":dbl[], "coeffs for intensity adjust":dbl[]}
  T4 = cluster{"xy cut pos correct":dbl[][], "3D reconst config":cluster{"xyz pos":u16[], "color 4":cluster{"color array":u32[], "num of colors":i32, "max":dbl, "min":dbl}, "autogain":bool, "zoom":dbl, "slice(T)/stack(F)":bool, "xy cut mag":dbl, "xy cut ofst":dbl, "z/xy comp":dbl, "y shift comp":dbl, "max plot":bool, "oblique angle [deg]":dbl, "voxel size z [um]":dbl, "voxel size xy[um]":dbl, "reverse v":bool, "reverse h":bool, "3D reconstruction":bool, "reverse z":bool}, "xy cut pos":dbl[][], "AOD scan speed ratio":dbl, "Nx":dbl, "stack method":enum16{"0pad to z", "0pad to x", "0pad to x and rot"}, "y shift":i32}
  T5 = cluster{"colors 2":cluster{"color array":u32[], "num of colors":i32, "max":dbl, "min":dbl}[], "on/off 2":bool[], "fast/slow":bool, "on/off":bool}
  T6 = enum16{"0pad to z", "0pad to x", "0pad to x and rot"}
  T7 = cluster{"xyz pos":u16[], "color 4":cluster{"color array":u32[], "num of colors":i32, "max":dbl, "min":dbl}, "autogain":bool, "zoom":dbl, "slice(T)/stack(F)":bool, "xy cut mag":dbl, "xy cut ofst":dbl, "z/xy comp":dbl, "y shift comp":dbl, "max plot":bool, "oblique angle [deg]":dbl, "voxel size z [um]":dbl, "voxel size xy[um]":dbl, "reverse v":bool, "reverse h":bool, "3D reconstruction":bool, "reverse z":bool}
  T8 = cluster{"img scan pos":dbl[][], "g1 disp [um]":dbl, "z spacing [um]":dbl, "g2 disp [pixels]":dbl, "scape scan pos ":dbl[]}
  T9 = cluster{"config cluster":cluster{"xy cut pos correct":dbl[][], "3D reconst config":cluster{"xyz pos":u16[], "color 4":cluster{"color array":u32[], "num of colors":i32, "max":dbl, "min":dbl}, "autogain":bool, "zoom":dbl, "slice(T)/stack(F)":bool, "xy cut mag":dbl, "xy cut ofst":dbl, "z/xy comp":dbl, "y shift comp":dbl, "max plot":bool, "oblique angle [deg]":dbl, "voxel size z [um]":dbl, "voxel size xy[um]":dbl, "reverse v":bool, "reverse h":bool, "3D reconstruction":bool, "reverse z":bool}, "xy cut pos":dbl[][], "AOD scan speed ratio":dbl, "Nx":dbl, "stack method":enum16{"0pad to z", "0pad to x", "0pad to x and rot"}, "y shift":i32}, "optimized param":dbl[][][][][], "volume indices":i32[]}
  T10 = cluster{"coeffs":cluster{"coeffs for r adjust":dbl[], "coeffs for x pos adjust":dbl[], "coeffs for intensity adjust":dbl[]}[], "config for coeffs":cluster{"# of avg for single waveform":u16, "skip [us]":dbl, "Nzf*Nv":i32, "ofst":dbl, "# of avg for volumes":u16, "limit data length":bool, "num of frames":i32, "Nv":i32}}
  T11 = enum16{"open", "replace", "create", "open or create", "replace or create", "replace or create with confirmation"}
  T12 = cluster{"img scan tangent":dbl[][], "img scan voltage":dbl[][]}
  T13 = cluster{"# of avg for single waveform":u16, "skip [us]":dbl, "Nzf*Nv":i32, "ofst":dbl, "# of avg for volumes":u16, "limit data length":bool, "num of frames":i32, "Nv":i32}
  T14 = cluster{"coeffs for r adjust":dbl[], "coeffs for x pos adjust":dbl[], "coeffs for intensity adjust":dbl[]}[]
  T15 = enum8{"Enabled", "Disabled", "Disabled and Grayed Out"}
  T16 = typedef "IMAQ AVI2 Refnum.ctl" = refnum<k20>
  T17 = typedef "Image Type" = u32
  T18 = typedef "IMAQ Image.ctl" = refnum<image>
  T19 = cluster{"color array":u32[], "num of colors":i32, "max":dbl, "min":dbl}[]
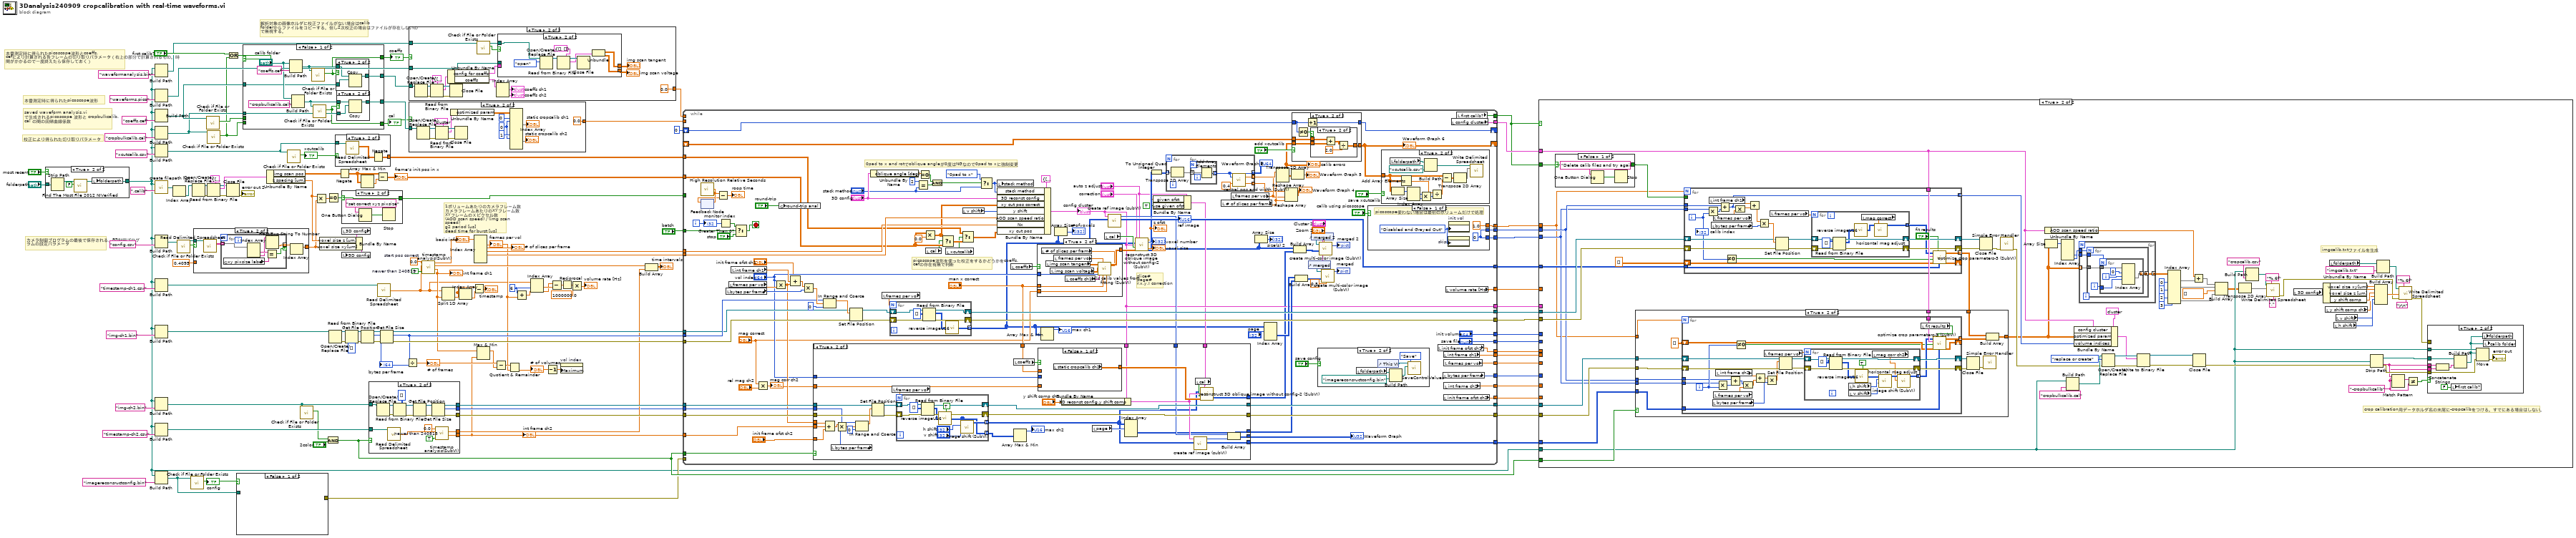
[diagram p0: block diagram]
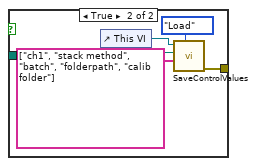
[diagram p2: hidden frame]
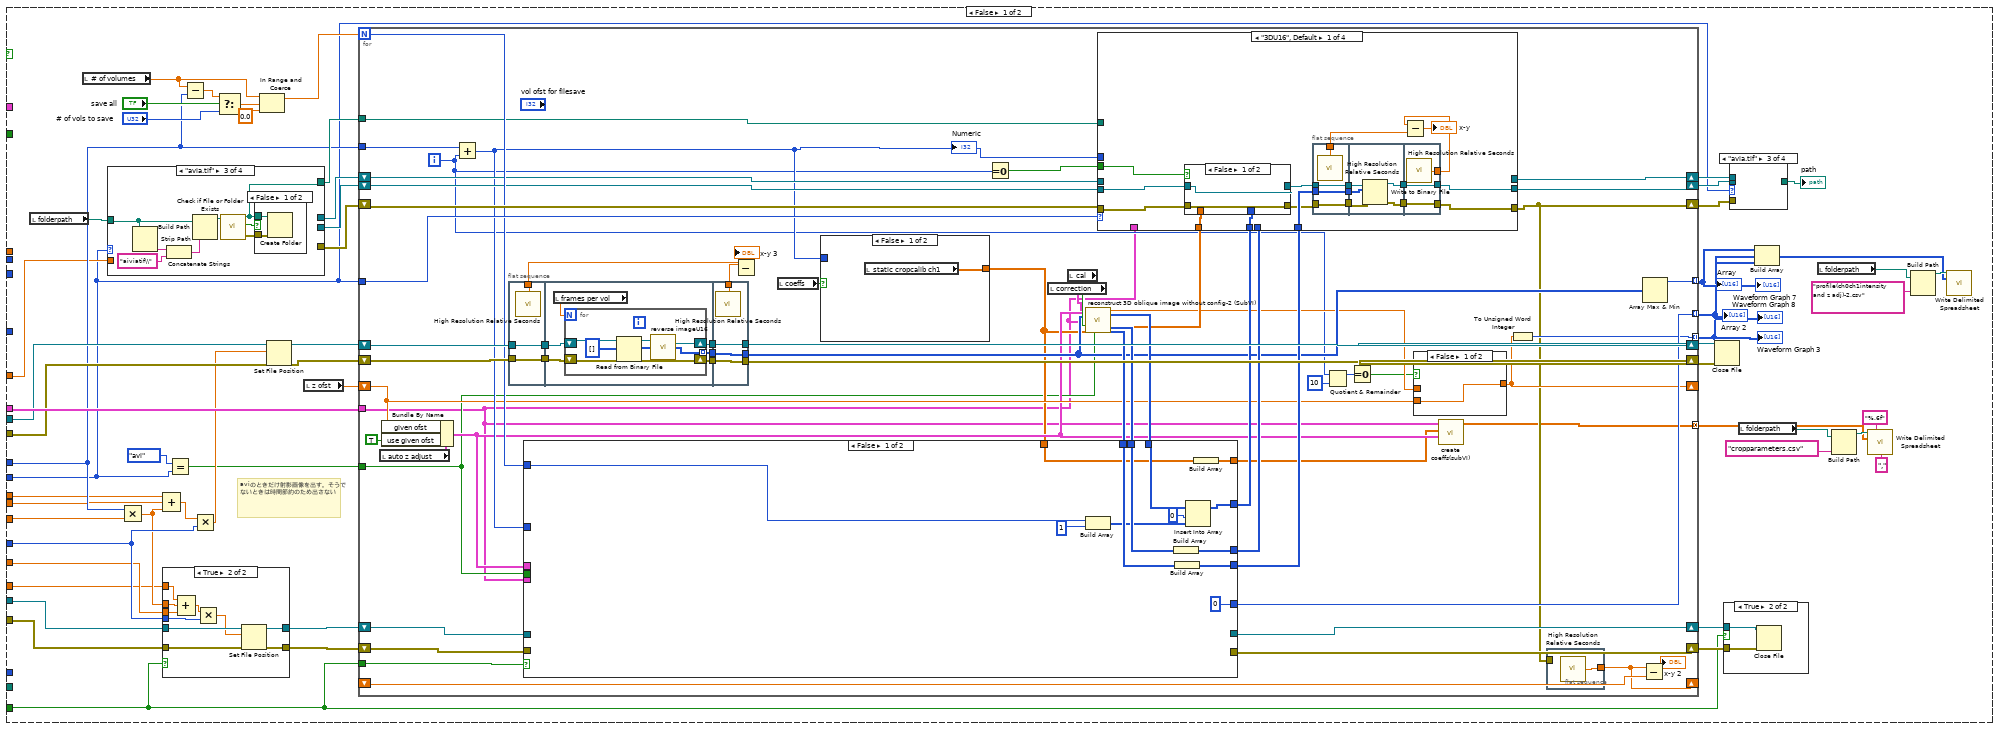
[diagram p3: hidden frame]
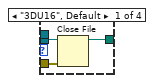
[diagram p6: hidden frame]
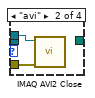
[diagram p7: hidden frame]
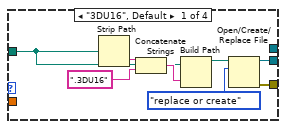
[diagram p9: hidden frame]
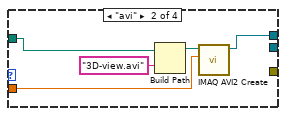
[diagram p10: hidden frame]
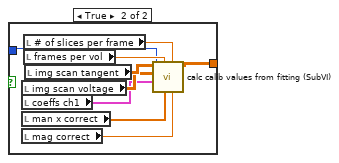
[diagram p13: hidden frame]
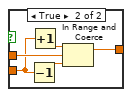
[diagram p14: hidden frame]
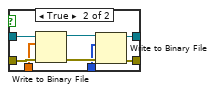
[diagram p15: hidden frame]
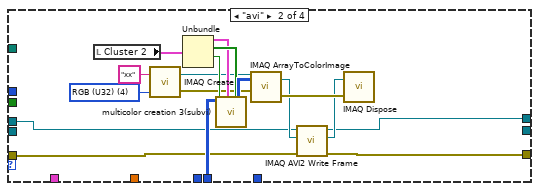
[diagram p16: hidden frame]
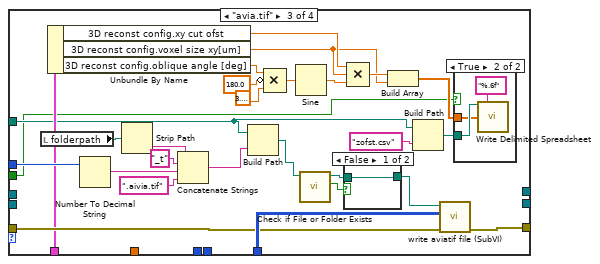
[diagram p17: hidden frame]
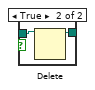
[diagram p18: hidden frame]
diagram:
  w3 = 6 ("index")
  w34 = TRUE  # newer than 240815
  w60 = 0.0  # start pos correct
  # "本番測定時に得られたpicoscope波形とcoeffs.cefにより計算される各フレームの切り取りパラメータ（右上の部分で計算されるもの。時間がかかるので一度終えたら保存しておく）"
  # "本番測定時に得られたpicoscope波形"
  # "saved waveform analysis.vi で生成されるpicoscope 波形と cropbulkcalib.cal の間の回帰曲線係数"
  # "校正により得られた切り取りパラメータ"
  # "カメラ制御プログラムの最後で保存される、FG制御プログラムの設定パラメータ"
  # "解析対象の画像ホルダに校正ファイルがない場合はcalib folderからファイルをコピーする。但し2次校正の場合はファイルが存在しないので無視する。"
  # "1ボリュームあたりのカメラフレーム数\nカメラフレームあたりのXYフレーム数\nXYフレームのＸピクセル数\n(AOD scan speed) / (img scan speed)\ng2 period [us]\ndead time for burst [us]"
  n1 = case shown="True" "most recent" {
    tunnel: "folderpath" -> [w132 w135]
    tunnel: [w132 w133] -> w16
    frame False {
    }
    frame True {
      n2 = Strip Path(path=w135) -> (stripped path=w134:path)  [unwired: 1 out]
      n3 = call "Find The Most File 2012 NIVerified.vi"("file(T)/folder(F)"=FALSE, "Folder Path In"=w134) -> ("File Path Out"=w133:path)  [unwired: 8 in, 1 out]
      n4 = local write "folderpath"(w133) -> ()
    }
  }
  n5 = Build Path(base path=w16, name or relative path="waveformanalysis.bin") -> (appended path=w15:path)
  n6 = Build Path(base path=w16, name or relative path="waveforms.pico") -> (appended path=w68:path)
  n7 = Build Path(base path=w16, name or relative path="coeffs.cef") -> (appended path=w59:path)
  n8 = Build Path(base path=w16, name or relative path="cropbulkcalib.cal") -> (appended path=w48:path)
  n9 = Build Path(base path=w16, name or relative path="xcutcalib.csv") -> (appended path=w63:path)
  n10 = call "create filepath list.vi"("regular expression"=".calib", "folder path (not file)"=w16) -> ("Array"=w130:path[])
  n11 = Build Path(base path=w16, name or relative path="config.csv") -> (appended path=w51:path)
  n12 = Build Path(base path=w16, name or relative path="timestamp-ch1.csv") -> (appended path=w121:path)
  n13 = Build Path(base path=w16, name or relative path="img-ch1.bin") -> (appended path=w120:path)
  n14 = Build Path(base path=w16, name or relative path="img-ch2.bin") -> (appended path=w122:path)
  n15 = Build Path(base path=w16, name or relative path="timestamp-ch2.csv") -> (appended path=w123:path)
  n16 = Build Path(base path=w16, name or relative path="imagereconsructconfig.bin") -> (appended path=w19:path)
  n17 = Index Array(array=w130) -> (element=w119:path)  [unwired: 1 in]
  n18 = call <vilib>:"Check if File or Folder Exists.vi"("path"=w51) -> ("file or folder exists?"=w53:bool)  [unwired: 8 in, 2 out]
  n19 = call <vilib>:"Check if File or Folder Exists.vi"("path"=w19) -> ("file or folder exists?"=w21:bool)  [unwired: 8 in, 2 out]
  "config" <- w21
  n20 = Open/Create/Replace File(file path (use dialog)=w119) -> (refnum out=w89:refnum<file>, error out=w95:errorcluster)  [unwired: 5 in, 1 out]
  n21 = case shown="True" w53 {
    tunnel: w51 -> [_ w139]
    tunnel: [w137 w138] -> w41
    tunnel: 0.4095 ("Numeric") -> [w137 _]
    frame False {
    }
    frame True {
      n22 = call-poly <vilib>:"Read Delimited Spreadsheet.vi"("file path (dialog if empty)"=w139) -> ("all rows"=w141:string[][])  [unwired: 9 in, 5 out]
      n23 = for {
        tunnel: w141 -> [w147] mode=indexing
        tunnel: [w144] -> w140 mode=indexing if=w143
        n24 = global read "filepath global variable.vi" "xy pixsize label"() -> (w142:string)
        n25 = Index Array(array=w147) -> (element #1=w146:string, element #2=w145:string)  [unwired: 2 in]
        n26 = Equal?(x=w146, y=w142) -> (x = y?=w143:bool)
        n27 = Fract/Exp String To Number(string=w145) -> (number=w144:dbl)  [unwired: 3 in, 1 out]
      }
      n28 = Index Array(array=w140) -> (element=w138:dbl)  [unwired: 1 in]
    }
  }
  n29 = call <vilib>:"Check if File or Folder Exists.vi"("path"=w59) -> ("file or folder exists?"=w55:bool)  [unwired: 8 in, 2 out]
  n30 = call <vilib>:"Check if File or Folder Exists.vi"("path"=w48) -> ("file or folder exists?"=w44:bool)  [unwired: 8 in, 2 out]
  n31 = Read from Binary File(5:T8 {"img scan pos"=[], "g1 disp [um]"=0.0, "z spacing [um]"=0.0, "g2 disp [pixels]"=0.0, "scape scan pos "=[]} ("calib values"), 8:w95, 11:w89) -> (0:w94:errorcluster, 2:w92:T8, 3:w88:refnum<file>)  [unwired: 3 in, 1 out]
  n32 = Close File(refnum=w88, error in=w94) -> (error out=→"error out 2":errorcluster)  [unwired: 1 out]
  n33 = Or(x="first calib?", y=w44) -> (x .or. y?=w57:bool)
  n34 = case shown="False" w21 {
    tunnel: w19 -> [_ w150]
    tunnel: [_ w149] -> w18
    frame False {
    }
    frame True {
      n35 = control-ref of="This VI"() -> (w151:refnum<vi>)
      n36 = call "SaveControlValues.vi"("Mode"=enum16{"Save", "Load"}."Load" ("Save Control Values Mode"), "exception list"=string[] ["ch1", "stack method", "batch", "folderpath", "calib folder"], "file path"=w150, "Target VI"=w151) -> ("error out"=w149:errorcluster)  [unwired: 1 in, 6 out]
    }
  }
  n37 = case shown="False" w57 {
    tunnel: w59 -> [w160 w173]
    tunnel: [w159 w173] -> w58
    tunnel: w55 -> [_ w172]
    tunnel: [w156 w172] -> w54
    tunnel: w48 -> [w158 w171]
    tunnel: [w155 w171] -> w46
    tunnel: [w153 w170] -> w45
    tunnel: w44 -> [_ w170]
    frame False {
      n38 = Build Path(base path="calib folder", name or relative path="coeffs.cef") -> (appended path=w157:path)
      n39 = Build Path(base path="calib folder", name or relative path="cropbulkcalib.cal") -> (appended path=w154:path)
      n40 = call <vilib>:"Check if File or Folder Exists.vi"("path"=w157) -> ("file or folder exists?"=w156:bool)  [unwired: 8 in, 2 out]
      n41 = call <vilib>:"Check if File or Folder Exists.vi"("path"=w154) -> ("file or folder exists?"=w153:bool)  [unwired: 8 in, 2 out]
      n42 = case shown="True" w156 {
        tunnel: w160 -> [_ w169]
        tunnel: [_ w168] -> w159
        tunnel: w157 -> [_ w167]
        frame False {
        }
        frame True {
          n43 = Copy(10:w169, 11:w167) -> (3:w168:path)  [unwired: 3 in, 2 out]
        }
      }
      n44 = case shown="True" w153 {
        tunnel: w154 -> [_ w166]
        tunnel: w158 -> [_ w165]
        tunnel: [_ w164] -> w155
        frame False {
        }
        frame True {
          n45 = Copy(10:w165, 11:w166) -> (3:w164:path)  [unwired: 3 in, 2 out]
        }
      }
    }
    frame True {
    }
  }
  "coeffs" <- w54
  "cal" <- w45
  n46 = Unbundle By Name(w92) -> ("img scan pos"=w23:dbl[][], "z spacing [um]"=w42:dbl)
  n47 = call <vilib>:"Check if File or Folder Exists.vi"("path"=w63) -> ("file or folder exists?"=w62:bool)  [unwired: 8 in, 2 out]
  "xcutcalib" <- w62
  n48 = call <vilib>:"Check if File or Folder Exists.vi"("path"=w122) -> ("file or folder exists?"=w81:bool)  [unwired: 8 in, 2 out]
  n49 = Multiply(x=w42, y=w41) -> (x*y=w40:dbl)
  n50 = And(x=w81, y="2color") -> (x .and. y?=w76:bool)
  n51 = Equal To 0?(x=w40) -> (x = 0?=w39:bool)
  n52 = Open/Create/Replace File(file path (use dialog)=w120) -> (refnum out=w113:refnum<file>, error out=w106:errorcluster)  [unwired: 5 in, 1 out]
  n53 = case shown="True" w62 {
    tunnel: w63 -> [_ w176]
    tunnel: [_ w174] -> w61
    frame False {
    }
    frame True {
      n54 = call-poly <vilib>:"Read Delimited Spreadsheet.vi"("file path (dialog if empty)"=w176) -> ("all rows"=w175:dbl[][])  [unwired: 9 in, 5 out]
      n55 = Negate(x=w175) -> (-x=w174:dbl[][])
    }
  }
  n56 = Negate(x=w23) -> (-x=w82:dbl[][])
  n57 = case shown="True" w39 {
    selector: w39 -> [w177 w178]
    tunnel: [w177 w178] -> w38
    frame False {
    }
    frame True {
      n58 = One Button Dialog(message="set correct xyz pixsize") -> (true=w179:bool)  [unwired: 1 in]
      n59 = Stop(stop? (T)=w179) -> ()
    }
  }
  n60 = local read "3D config"() -> (w91:T7)
  n61 = Bundle By Name(cluster=w91, "voxel size z [um]"=w42, "voxel size xy[um]"=w41) -> (w90:T7)
  n62 = local write "3D config"(w90) -> ()
  n63 = Read from Binary File(5:u16[][] [], 8:w106, 11:w113) -> (0:w107:errorcluster, 3:w112:refnum<file>)  [unwired: 3 in, 2 out]
  n64 = Get File Position(4:w107, 7:w112) -> (0:w108:errorcluster, 2:w105:i64, 3:w111:refnum<file>)
  "bytes per frame" <- w105
  n65 = Array Max & Min(array=w82) -> (min value=w118:dbl)  [unwired: 3 out]
  n66 = case shown="True" w76 {
    tunnel: [_ w187] -> w86
    tunnel: [_ w190] -> w103
    tunnel: [_ w189] -> w102
    tunnel: [_ w186] -> w99
    tunnel: [_ w185] -> w98
    tunnel: w122 -> [_ w184]
    tunnel: w123 -> [_ w183]
    frame False {
    }
    frame True {
      w181 = TRUE  # newer than 240815
      n67 = Open/Create/Replace File(file path (use dialog)=w184) -> (refnum out=w196:refnum<file>, error out=w197:errorcluster)  [unwired: 5 in, 1 out]
      n68 = call-poly <vilib>:"Read Delimited Spreadsheet.vi"("file path (dialog if empty)"=w183) -> ("first row"=w188:dbl[])  [unwired: 9 in, 5 out]
      n69 = Read from Binary File(5:u16[][] [], 8:w197, 11:w196) -> (0:w192:errorcluster, 3:w193:refnum<file>)  [unwired: 3 in, 2 out]
      n70 = Get File Position(4:w192, 7:w193) -> (0:w194:errorcluster, 3:w191:refnum<file>)  [unwired: 1 out]
      n71 = Get File Size(file=w191, error in=w194) -> (refnum out=w190:refnum<file>, size (in bytes)=w185:i64, 0:w189:errorcluster)
      n72 = call "timestamp analysis(SubVI).vi"("newer than 240815"=w181, "first row"=w188, "start pos correct"=0.0) -> ("Numeric"=w187:dbl, "Array"=w186:dbl[])  [unwired: 6 in, 1 out]
    }
  }
  "int frame ch2" <- w86
  n73 = Subtract(x=w82, y=w118) -> (x-y=w101:dbl[][])
  "frame's init pos in x" <- w101
  n74 = call-poly <vilib>:"Read Delimited Spreadsheet.vi"("file path (dialog if empty)"=w121) -> ("first row"=w5:dbl[])  [unwired: 9 in, 5 out]
  n75 = Get File Size(file=w111, error in=w108) -> (refnum out=w110:refnum<file>, size (in bytes)=w104:i64, 0:w109:errorcluster)
  n76 = Divide(x=w104, y=w105) -> (x/y=w87:dbl)
  "# of frames" <- w87
  n77 = case shown="True" w45 {
    tunnel: w46 -> [_ w208]
    tunnel: [_ 0.0 ("mean")] -> w47
    frame False {
    }
    frame True {
      w200 = 0 ("disabled index (vol)")
      n78 = Open/Create/Replace File(file path (use dialog)=w208) -> (refnum out=w207:refnum<file>, error out=w211:errorcluster)  [unwired: 5 in, 1 out]
      n79 = Read from Binary File(5:T9 {"config cluster"={"xy cut pos correct"=[], "3D reconst config"={"xyz pos"=[], "color 4"={"color array"=[], "num of colors"=0, "max"=0.0, "min"=0.0}, "autogain"=FALSE, "zoom"=0.0, "slice(T)/stack(F)"=FALSE, "xy cut mag"=0.0, "xy cut ofst"=0.0, "z/xy comp"=0.0, "y shift comp"=0.0, "max plot"=FALSE, "oblique angle [deg]"=0.0, "voxel size z [um]"=0.0, "voxel size xy[um]"=0.0, "reverse v"=FALSE, "reverse h"=FALSE, "3D reconstruction"=FALSE, "reverse z"=FALSE}, "xy cut pos"=[], "AOD scan speed ratio"=0.0, "Nx"=0.0, "stack method"=enum."0pad to z", "y shift"=0}, "optimized param"=[], "volume indices"=[]} ("cluster"), 8:w211, 11:w207) -> (0:w210:errorcluster, 2:w204:T9, 3:w209:refnum<file>)  [unwired: 3 in, 1 out]
      n80 = Unbundle By Name(w204) -> ("optimized param"=w203:dbl[][][][][])
      n81 = Close File(refnum=w209, error in=w210) -> ()  [unwired: 2 out]
      n82 = Index Array(array=w203, index (dim 0) #1=0 ("index (dim 5)"), index (dim 1) #1=w200, index (dim 0) #2=1 ("index (dim 5)"), index (dim 1) #2=w200) -> (element #1=→"static cropcalib ch1":dbl[][][], element #2=→"static cropcalib ch2":dbl[][][])  [unwired: 6 in]
    }
  }
  n83 = case shown="True" w54 {
    tunnel: w58 -> [_ w226]
    tunnel: w68 -> [_ w224]
    tunnel: [_ 0.0 ("mean")] -> w67
    tunnel: w15 -> [_ w213]
    frame False {
    }
    frame True {
      n84 = Open/Create/Replace File(file path (use dialog)=w226) -> (refnum out=w225:refnum<file>, error out=w229:errorcluster)  [unwired: 5 in, 1 out]
      n85 = Read from Binary File(5:T10 {"coeffs"=[], "config for coeffs"={"# of avg for single waveform"=0, "skip [us]"=0.0, "Nzf*Nv"=0, "ofst"=0.0, "# of avg for volumes"=0, "limit data length"=FALSE, "num of frames"=0, "Nv"=0}}, 8:w229, 11:w225) -> (0:w228:errorcluster, 2:w219:T10, 3:w227:refnum<file>)  [unwired: 3 in, 1 out]
      n86 = Unbundle By Name(w219) -> ("config for coeffs"=w218:T13, "coeffs"=w217:T14)
      n87 = Close File(refnum=w227, error in=w228) -> ()  [unwired: 2 out]
      n88 = call <vilib>:"Check if File or Folder Exists.vi"("path"=w213) -> ("file or folder exists?"=w212:bool, "dup path"=w214:path)  [unwired: 8 in, 1 out]
      n89 = Index Array(array=w217) -> (element #1=→"coeffs ch1":T3, element #2=→"coeffs ch2":T3)  [unwired: 2 in]
      n90 = case shown="True" w212 {
        tunnel: w224 -> [w240 _]
        tunnel: w218 -> [w239 _]
        tunnel: [w232 w243] -> w216
        tunnel: [w231 w242] -> w215
        tunnel: w214 -> [w230 w241]
        frame False {
          n91 = call "extract galvo voltage readout clusterinput (SubVI).vi"("file path (use dialog)"=w240, "cluster"=w239) -> ("img scan tangent"=w232:dbl[][], "img scan voltage"=w231:dbl[][])  [unwired: 7 in, 5 out]
          n92 = Bundle("img scan tangent"=w232, "img scan voltage"=w231) -> (w238:T12)  [unwired: 1 in]
          n93 = Open/Create/Replace File(file path (use dialog)=w230, operation (0:open)=T11."replace or create") -> (refnum out=w236:refnum<file>, error out=w233:errorcluster)  [unwired: 4 in, 1 out]
          n94 = Write to Binary File(file (use dialog)=w236, data=w238, error in=w233) -> (refnum out=w237:refnum<file>, error out=w234:errorcluster)  [unwired: 3 in, 1 out]
          n95 = Close File(refnum=w237, error in=w234) -> ()  [unwired: 2 out]
        }
        frame True {
          n96 = Open/Create/Replace File(file path (use dialog)=w241, operation (0:open)=T11."open") -> (refnum out=w246:refnum<file>)  [unwired: 4 in, 2 out]
          n97 = Read from Binary File(5:T12 {"img scan tangent"=[], "img scan voltage"=[]} ("output cluster"), 11:w246) -> (2:w245:T12, 3:w247:refnum<file>)  [unwired: 4 in, 2 out]
          n98 = Close File(refnum=w247) -> ()  [unwired: 1 in, 2 out]
          n99 = Unbundle(w245) -> ("img scan tangent"=w243:dbl[][], "img scan voltage"=w242:dbl[][])
        }
      }
      "img scan tangent" <- w216
      "img scan voltage" <- w215
    }
  }
  n100 = call "timestamp analysis(SubVI).vi"("newer than 240815"=w34, "first row"=w5, "start pos correct"=w60) -> ("Numeric"=w85:dbl, "Array"=w32:dbl[], "Array 2"=w117:dbl[])  [unwired: 6 in]
  "basic info" <- w117
  "int frame ch1" <- w85
  n101 = Split 1D Array(array=w5, index=w85) -> (second subarray=w33:dbl[])  [unwired: 1 out]
  n102 = Index Array(array=w33) -> (element=w97:dbl)  [unwired: 1 in]
  n103 = Subtract(x=w33, y=w97) -> (x-y=→"timestamp":dbl[])
  n104 = Index Array(array=w117) -> (element #1=w12:dbl, element #2=→"# of slices per frame":dbl, element #3=w116:dbl, element #4=w115:dbl)  [unwired: 6 in, 2 out]
  "frames per vol" <- w12
  n105 = Max & Min(x=w85, y=w86) -> (max(x,y)=w84:dbl)  [unwired: 1 out]
  n106 = Subtract(x=w87, y=w84) -> (x-y=w83:dbl)
  n107 = Quotient & Remainder(x=w83, y=w12) -> (floor(x/y)=w79:dbl)  [unwired: 1 out]
  "# of volumes" <- w79
  n108 = Add(x=w3, y=w12) -> (x+y=w4:dbl)
  n109 = Index Array(array=w5, index #1=w3, index #2=w4) -> (element #1=w11:dbl, element #2=w10:dbl)
  n110 = Decrement(x=w79) -> (x-1=w78:dbl)
  n111 = Subtract(x=w10, y=w11) -> (x-y=w9:dbl)
  n112 = property on="vol index" class="DigNum (strict)"("Maximum"=w78) -> ()  [unwired: 2 in, 2 out]
  n113 = Reciprocal(x=w9) -> (1/x=w7:dbl)
  n114 = Multiply(x=w7, y=1000000.0) -> (x*y=→"volume rate [Hz]":dbl)
  n115 = Build Array(w32, w99) -> (→"time intervals":dbl[][])
  n116 = while {
    tunnel: w102 -> [w366]
    tunnel: w109 -> [w367]
    tunnel: w110 -> [w368]
    tunnel: [w364] -> w72
    tunnel: [w363] -> w77
    tunnel: [w359] -> w74
    tunnel: [w358] -> w73
    tunnel: w86 -> [w276]
    tunnel: w116 -> [w331]
    tunnel: w115 -> [w332]
    tunnel: w104 -> [w369]
    tunnel: w103 -> [w365]
    tunnel: w101 -> [w326]
    tunnel: w76 -> [w362]
    tunnel: w98 -> [w356]
    tunnel: [w333] -> w50
    tunnel: [w330] -> w71
    tunnel: [w329] -> w70
    tunnel: w67 -> [_]
    shift-right: [w303] -> _
    shift-left: _ -> [w307]
    shift-right: [w305] -> _
    shift-left: 0 -> [w306]
    tunnel: w61 -> [w301]
    tunnel: [w296] -> w30
    tunnel: w47 -> [_]
    tunnel: w38 -> [_]
    tunnel: [w291] -> w37
    tunnel: [w290] -> w36
    tunnel: [w289] -> w35
    tunnel: [w287] -> w31
    tunnel: ["init volume"] -> w29
    tunnel: ["save file"] -> w28
    tunnel: [w280] -> w27
    tunnel: [w279] -> w26
    tunnel: [w278] -> w25
    tunnel: [w277] -> w24
    tunnel: w18 -> [_]
    tunnel: [w271] -> w14
    tunnel: [w270] -> w13
    tunnel: "batch" -> [w266]
    tunnel: [w264] -> w1
    i -> [w269]
    stop <- w265 stop-if-true
    # "0pad to x and rotでoblique angleが0度はNGなので0pad to xに強制変更"
    # "picoscope波形を使った校正をするかどうかをcoeffs.cefの存在有無で判断"
    # "slice#\npage#\nr,x,y,I correction"
    n117 = call <vilib>:"High Resolution Relative Seconds.vi"() -> ("relative seconds"=w350:dbl)
    n118 = feedback-in #1(w350) -> ()
    n119 = feedback #1() -> (w349:dbl)  [unwired: 1 in]
    n120 = Subtract(x=w350, y=w349) -> (x-y=→"roop time":dbl)
    n121 = Greater Than 0?(x=w269) -> (x > 0?=w268:bool)
    n122 = local read "bytes per frame"() -> (w354:i64)
    n123 = local read "frames per vol"() -> (w357:dbl)
    n124 = local read "int frame ch1"() -> (w352:dbl)
    n125 = Select(t=w268, s=w266, f="stop") -> (s? t:f=w265:bool)
    n126 = Multiply(x="mag correct", y="rel mag ch2") -> (x*y=w319:dbl)
    "mag corr ch2" <- w319
    n127 = Multiply(x="vol index", y=w357) -> (x*y=w353:dbl)
    n128 = global write "global for picoscope.vi" "round-trip anal"("round-trip") -> ()
    n129 = Compound Arithmetic op=ADD("init frame ofst ch1", w352, w353) -> (w370:dbl)
    n130 = Multiply(x=w370, y=w354) -> (x*y=w373:dbl)
    n131 = In Range and Coerce(upper limit=w369, x=w373, lower limit=i64 0) -> (coerced(x)=w371:dbl)  [unwired: 1 out]
    n132 = Set File Position(offset (in bytes) (0)=w371, refnum=w368, error in=w367) -> (refnum out=w361:refnum<file>, error out=w360:errorcluster)  [unwired: 1 in]
    n133 = Unbundle By Name("3D config") -> ("oblique angle [deg]"=w258:dbl)
    n134 = local read "frames per vol"() -> (w355:dbl)
    n135 = for {
      N: w355 -> [_]
      tunnel: [w432] -> w261 mode=indexing
      shift-right: [w436] -> w359
      shift-left: w360 -> [w438]
      shift-right: [w435] -> w358
      shift-left: w361 -> [w437]
      n136 = Read from Binary File(5:u16[][] [], 8:w438, 11:w437) -> (0:w436:errorcluster, 2:w433:u16[][], 3:w435:refnum<file>)  [unwired: 3 in, 1 out]
      n137 = call "reverse imageU16.vi"("output array in"=w433) -> ("output array out"=w432:u16[][])  [unwired: 2 in]
    }
    n138 = Equal?(x=2, y="stack method") -> (x = y?=w256:bool)
    n139 = Equal To 0?(x=w258) -> (x = 0?=w257:bool)
    n140 = Multiply(x=w326, y=0.0) -> (x*y=w297:dbl[][])
    n141 = local read "cal"() -> (w292:bool)
    n142 = And(x=w257, y=w256) -> (x .and. y?=w255:bool)
    n143 = Select(t=w297, s=w292, f=w326) -> (s? t:f=w302:dbl[][])
    n144 = local read "xcutcalib"() -> (w300:bool)
    n145 = Select(t=w301, s=w300, f=w302) -> (s? t:f=w299:dbl[][])
    n146 = local read "v shift"() -> (w334:i32)
    n147 = Select(t=T6."0pad to x", s=w255, f="stack method") -> (s? t:f=w252:T6)
    n148 = local write "stack method"(w252) -> ()
    n149 = Bundle By Name(cluster=T4 {"xy cut pos correct"=[[0.0, 0.0, 0.0, -7.0], [0.0, 0.0, 0.0, -7.0], [0.0, 0.0, 0.0, -7.0], [0.0, 0.0, 0.0, -7.0], [0.0, 0.0, 0.0, -7.0], [0.0, 0.0, 0.0, 0.0], [0.0, 0.0, 0.0, 0.0], [0.0, 0.0, 0.0, 0.0], [0.0, 0.0, 0.0, 0.0], [0.0, 0.0, 0.0, 0.0]], "3D reconst config"={"xyz pos"=[271, 288, 150], "color 4"={"color array"=[0, 8388736, 16711680, 16776960, 16776960, 16711680, 16448250, 16448250], "num of colors"=4, "max"=7000.900000000023, "min"=100.0}, "autogain"=TRUE, "zoom"=1.0, "slice(T)/stack(F)"=FALSE, "xy cut mag"=1.0000000000000004, "xy cut ofst"=0.0, "z/xy comp"=0.9999999999999998, "y shift comp"=0.0, "max plot"=TRUE, "oblique angle [deg]"=45.0, "voxel size z [um]"=5.066639031844781, "voxel size xy[um]"=0.455, "reverse v"=FALSE, "reverse h"=TRUE, "3D reconstruction"=TRUE, "reverse z"=FALSE}, "xy cut pos"=[[0.0, 4.540011367701254, 4.853687897950067, 5.137490472936861], [207.4696403005795, 211.47606963402166, 212.00384284364657, 211.78310750754565], [421.4617608333166, 425.35948216288944, 425.8192091410847, 426.1901440855853], [642.40206546069, 646.4425179098467, 646.8897974066831, 647.0541041606228], [871.5767939231397, 875.391532043652, 875.6172463722967, 876.1035279773913], [1108.4465553617717, 1112.4031947697777, 1112.9766087443859, 1112.9317978114932], [1350.135151750549, 1354.1980096661523, 1354.7506778384952, 1354.8104257490188], [1587.7666990483574, 1591.187266925832, 1591.5457543889736, 1591.7075716466416], [1812.700155695724, 1816.1970681255343, 1816.7497362978775, 1816.9289800294482], [2008.714793817587, 2011.9801830941183, 2012.2158554078503, 2013.1535656702342]], "AOD scan speed ratio"=5.0, "Nx"=224.4, "stack method"=enum."0pad to z", "y shift"=-6} ("config in"), "stack method"=w252, "3D reconst config"="3D config", "xy cut pos correct"=w297, "y shift"=w334, "AOD scan speed ratio"=w332, "Nx"=w331, "xy cut pos"=w299) -> (w287:T4)
    "config cluster" <- w287
    n150 = local read "coeffs"() -> (w294:bool)
    n151 = case shown="True" w294 {
      tunnel: [w388 w394] -> w328
      tunnel: "vol index" -> [_ w391]
      tunnel: "man x correct" -> [_ w390]
      tunnel: "mag correct" -> [_ w389]
      frame False {
        n152 = local read "static cropcalib ch1"() -> (w388:dbl[][][])
      }
      frame True {
        n153 = local read "# of slices per frame"() -> (w392:dbl)
        n154 = local read "img scan tangent"() -> (w395:dbl[][])
        n155 = local read "img scan voltage"() -> (w396:dbl[][])
        n156 = local read "frames per vol"() -> (w393:dbl)
        n157 = local read "coeffs ch1"() -> (w397:T3)
        n158 = call "calc calib values from fitting (SubVI).vi"("mag correct"=w389, "# of slices"=w392, "man x correct"=w390, "# of pages"=w393, "volume index"=w391, "Cluster"=w397, "img scan voltage"=w396, "img scan tangent"=w395) -> ("Array"=w394:dbl[][][])  [unwired: 3 in]
      }
    }
    n159 = Array Max & Min(array=w261) -> (max value=→"max ch1":u16)  [unwired: 3 out]
    n160 = Array Size(array=w261) -> (size(s)=→"#ofvoxels":i32[])
    n161 = local read "cal"() -> (w293:bool)
    n162 = call "create ref image (subVI).vi"("Array in"=w261, "config in"=w287) -> ("ref image"=w330:u16[][], "Waveform Graph"=w324:u32[])  [unwired: 8 in]
    "ref image" <- w330
    n163 = call "reconstruct 3D oblique image without config-2 (SubVI).vi"("correction"="correction", "auto z adjust"="auto z adjust", "image in"=w261, "config in"=w287, "cropcalib"=w293, "cropcalib data"=w328) -> ("voxel number"=→"voxel number":i32[], "z ofst"=w282:dbl, "voxel size [um]"=→"voxel size":dbl[], "combined img"=w250:u16[][], "xyz"=w318:u16[][][])  [unwired: 2 in, 3 out]
    "z ofst" <- w282
    n164 = To Unsigned Quad Integer(1:w318) -> (0:w316:u64[][][])
    n165 = Bundle By Name(cluster="auto z adjust", "given ofst"=w282, "use given ofst"=TRUE) -> (w281:T2)
    n166 = case shown="True" w362 {
      tunnel: w276 -> [_ w476]
      tunnel: w366 -> [_ w471]
      tunnel: w353 -> [_ w470]
      tunnel: w365 -> [_ w469]
      tunnel: [_ w466] -> w364
      tunnel: [_ w465] -> w363
      tunnel: w356 -> [_ w464]
      tunnel: [_ w461] -> w262
      tunnel: [_ w450] -> w341
      tunnel: w287 -> [_ w457]
      tunnel: [_ w460] -> w329
      tunnel: "vol index" -> [_ w458]
      tunnel: w324 -> [w440 w454]
      tunnel: [w439 w452] -> w323
      tunnel: w319 -> [_ w444]
      tunnel: "man x correct" -> [_ w451]
      tunnel: w281 -> [_ w446]
      tunnel: "init frame ofst ch2" -> [_ w445]
      frame False {
        n167 = Build Array(w440) -> (w439:u32[][])
      }
      frame True {
        n168 = Compound Arithmetic op=ADD(w470, w476, w445) -> (w473:dbl)
        n169 = local read "bytes per frame"() -> (w463:i64)
        n170 = Multiply(x=w473, y=w463) -> (x*y=w474:dbl)
        n171 = In Range and Coerce(upper limit=w464, x=w474, lower limit=i64 0) -> (coerced(x)=w472:dbl)  [unwired: 1 out]
        n172 = Set File Position(offset (in bytes) (0)=w472, refnum=w469, error in=w471) -> (refnum out=w467:refnum<file>, error out=w468:errorcluster)  [unwired: 1 in]
        n173 = local read "frames per vol"() -> (w447:dbl)
        n174 = for {
          N: w447 -> [_]
          tunnel: [w478] -> w442 mode=indexing
          shift-right: [w485] -> w466
          shift-left: w468 -> [w487]
          shift-right: [w484] -> w465
          shift-left: w467 -> [w486]
          tunnel: [w477] -> w441 mode=indexing
          n175 = Read from Binary File(5:u16[][] [], 8:w487, 11:w486) -> (0:w485:errorcluster, 2:w481:u16[][], 3:w484:refnum<file>)  [unwired: 3 in, 1 out]
          n176 = call "reverse imageU16.vi"("output array in"=w481, "reverse h"=TRUE ("reverse h 2")) -> ("output array out"=w477:u16[][])  [unwired: 1 in]
          n177 = call "image shift (SubVI).vi"("v shift"="v shift", "h shift"="h shift", "Array in"=w477) -> ("Array out"=w478:u16[][])  [unwired: 8 in]
        }
        n178 = local read "coeffs"() -> (w449:bool)
        n179 = Array Max & Min(array=w441) -> (max value=→"max ch2":u16)  [unwired: 3 out]
        n180 = case shown="False" w449 {
          tunnel: [w488 w492] -> w459
          tunnel: w458 -> [_ w491]
          tunnel: w451 -> [_ w490]
          tunnel: w444 -> [_ w489]
          frame False {
            n181 = local read "static cropcalib ch2"() -> (w488:dbl[][][])
          }
          frame True {
            n182 = local read "# of slices per frame"() -> (w493:dbl)
            n183 = local read "img scan tangent"() -> (w496:dbl[][])
            n184 = local read "img scan voltage"() -> (w495:dbl[][])
            n185 = local read "frames per vol"() -> (w497:dbl)
            n186 = local read "coeffs ch2"() -> (w494:T3)
            n187 = call "calc calib values from fitting (SubVI).vi"("mag correct"=w489, "# of slices"=w493, "man x correct"=w490, "# of pages"=w497, "volume index"=w491, "Cluster"=w494, "img scan voltage"=w495, "img scan tangent"=w496) -> ("Array"=w492:dbl[][][])  [unwired: 3 in]
          }
        }
        n188 = Bundle By Name(cluster=w457, "3D reconst config.y shift comp"="y shift comp ch2") -> (w455:T4)
        n189 = local read "page"() -> (w462:i32)
        n190 = Index Array(array=w442, index (dim 0)=w462) -> (element=w450:u16[][])  [unwired: 2 in]
        n191 = call "create ref image (subVI).vi"("Array in"=w442, "config in"=w455) -> ("ref image"=w460:u16[][], "Waveform Graph"=w453:u32[])  [unwired: 8 in]
        n192 = local read "cal"() -> (w448:bool)
        n193 = call "reconstruct 3D oblique image without config-2 (SubVI).vi"("auto z adjust"=w446, "image in"=w442, "config in"=w455, "cropcalib"=w448, "cropcalib data"=w459) -> ("combined img"=w461:u16[][])  [unwired: 3 in, 7 out]
        n194 = Build Array(w454, w453) -> (w452:u32[][])
      }
    }
    "Waveform Graph" <- w323
    n195 = for {
      tunnel: w316 -> [w429] mode=indexing
      tunnel: [w427] -> w317 mode=indexing
      tunnel: [w425] -> w315 mode=indexing
      tunnel: [w424] -> w312 mode=indexing
      n196 = Transpose 2D Array(2D array=w429) -> (transposed array=w428:u64[][])
      n197 = for {
        tunnel: w428 -> [w431] mode=indexing
        tunnel: [w430] -> w427 mode=indexing
        n198 = Add Array Elements(numeric array=w431) -> (sum=w430:u64)
      }
      n199 = call "central pos and width (SubVI).vi"("threshold level [0-1]"=0.4, "proj profile"=w427) -> ("width"=w424:dbl, "center pos"=w425:dbl)
    }
    "Waveform Graph 2" <- w317
    n200 = local read "# of slices per frame"() -> (w314:dbl)
    n201 = local read "frames per vol"() -> (w313:dbl)
    n202 = Array Size(array=w250) -> (size(s)=→"size(s) 2":i32[])
    n203 = Index Array(array=w261, index (dim 0)="page") -> (element=w295:u16[][])  [unwired: 2 in]
    n204 = Reshape Array(w315, w313, w314) -> (w308:dbl[][])
    "calib errors" <- w308
    n205 = Reshape Array(w312, w313, w314) -> (→"Waveform Graph 4":dbl[][])
    n206 = Transpose 2D Array(2D array=w308) -> (transposed array=→"Waveform Graph 5":dbl[][])
    n207 = case shown="True" "add xcutcalib" {
      tunnel: w308 -> [_ w417]
      tunnel: w307 -> [w411 w416]
      tunnel: [w411 w415] -> w303
      tunnel: w306 -> [w410 w412]
      tunnel: [w410 w414] -> w305
      frame False {
      }
      frame True {
        n208 = Not Equal To 0?(x=w412) -> (x != 0?=w413:bool)
        n209 = Increment(x=w412) -> (x+1=w414:i32)
        n210 = case shown="True" w413 {
          tunnel: w417 -> [w418 w423]
          tunnel: w416 -> [_ w422]
          tunnel: [w418 w419] -> w415
          frame False {
          }
          frame True {
            n211 = Add(x=w422, y=w423) -> (x+y=w420:dbl[][])
            n212 = Divide(x=w420, y=2.0) -> (x/y=w419:dbl[][])
          }
        }
      }
    }
    "Waveform Graph 6" <- w303
    n213 = Build Array(w250, w262) -> (w345:u16[][][])
    n214 = Build Array(w295, w341) -> (w343:u16[][][])
    n215 = control-ref of="merged"() -> (w340:refnum<vi>)
    n216 = control-ref of="merged 2"() -> (w347:refnum<vi>)
    n217 = case shown="True" "save config" {
      frame False {
      }
      frame True {
        n218 = local read "folderpath"() -> (w374:path)
        n219 = control-ref of="This VI"() -> (w378:refnum<vi>)
        n220 = Build Path(base path=w374, name or relative path=path "imagereconsructconfig.bin") -> (appended path=w376:path)
        n221 = call "SaveControlValues.vi"("Mode"=enum16{"Save", "Load"}."Save" ("Save Control Values Mode"), "file path"=w376, "Target VI"=w378) -> ()  [unwired: 2 in, 7 out]
      }
    }
    n222 = call "create multi-color image (SubVI).vi"("Zoom"="Zoom 2", "Array"=w345, "Cluster"="Cluster 2", "Picture in"=w347) -> ("new picture 2"=→"merged 2":picture)  [unwired: 7 in]
    n223 = call "create multi-color image (SubVI).vi"("Zoom"=sgl 0.5 ("Zoom 3"), "Array"=w343, "Cluster"="Cluster 2", "Picture in"=w340) -> ("new picture 2"=→"merged":picture)  [unwired: 7 in]
    n224 = case shown="False" "calib using picoscope" {
      tunnel: [w380 "init vol"] -> w291
      tunnel: [w380 "skip"] -> w290
      tunnel: [1.0 w383] -> w289
      frame False {
        w380 = 0 ("init vol")
        w379 = T15."Disabled and Grayed Out" ("Disabled")
        # "picoscope使わない場合は最初のボリュームだけで処理"
        n225 = property on="skip" class="DigNum (strict)"("DisabledEnum"=w379) -> ()  [unwired: 2 in, 2 out]
        n226 = property on="init vol" class="DigNum (strict)"("DisabledEnum"=w379) -> ()  [unwired: 2 in, 2 out]
      }
      frame True {
        w382 = T15."Enabled" ("Disabled")
        n227 = property on="skip" class="DigNum (strict)"("DisabledEnum"=w382) -> ()  [unwired: 2 in, 2 out]
        n228 = property on="init vol" class="DigNum (strict)"("DisabledEnum"=w382) -> ()  [unwired: 2 in, 2 out]
        n229 = local read "# of volumes"() -> (w384:dbl)
        n230 = Subtract(x=w384, y="init vol") -> (x-y=w385:dbl)
        n231 = Quotient & Remainder(x=w385, y="skip") -> (floor(x/y)=w383:dbl)  [unwired: 1 out]
      }
    }
    n232 = case shown="True" "save xcutcalib" {
      tunnel: w303 -> [_ w400]
      frame False {
      }
      frame True {
        n233 = local read "folderpath"() -> (w409:path)
        n234 = Array Size(array=w400) -> (size(s)=w406:i32[])
        n235 = Add Array Elements(numeric array=w400) -> (sum=w402:dbl)
        n236 = Index Array(array=w406) -> (element #1=w404:i32, element #2=w405:i32)  [unwired: 2 in]
        n237 = Multiply(x=w404, y=w405) -> (x*y=w403:i32)
        n238 = Build Path(base path=w409, name or relative path=path "xcutcalib.csv") -> (appended path=w407:path)
        n239 = Divide(x=w402, y=w403) -> (x/y=w401:dbl)
        n240 = Subtract(x=w400, y=w401) -> (x-y=w399:dbl[][])
        n241 = Transpose 2D Array(2D array=w399) -> (transposed array=w398:dbl[][])
        n242 = call-poly <vilib>:"Write Delimited Spreadsheet.vi"("file path (dialog if empty)"=w407, "2D data"=w398) -> ()  [unwired: 12 in, 2 out]
      }
    }
    n243 = local read "init frame ofst ch1"() -> (w270:dbl)
    n244 = local read "bytes per frame"() -> (w280:i64)
    n245 = local read "int frame ch1"() -> (w278:dbl)
    n246 = local read "init frame ofst ch2"() -> (w271:dbl)
    n247 = local read "frames per vol"() -> (w279:dbl)
    n248 = local read "int frame ch2"() -> (w277:dbl)
    n249 = local read "volume rate [Hz]"() -> (w264:dbl)
    n250 = local read "config cluster"() -> (w333:T4)
    n251 = local read "first calib?"() -> (w296:bool)
    "monitor index" <- w269
  }
  n252 = case shown="True" w30 {
    tunnel: w77 -> [w516 w922]
    tunnel: w76 -> [w513 w921]
    tunnel: w74 -> [w519 w901]
    tunnel: w73 -> [w521 w900]
    tunnel: w72 -> [w514 w899]
    tunnel: w71 -> [_ w896]
    tunnel: w70 -> [_ w895]
    tunnel: w30 -> [_ w894]
    tunnel: w50 -> [_ w888]
    tunnel: w16 -> [_ w887]
    tunnel: w37 -> [_ w886]
    tunnel: w36 -> [_ w885]
    tunnel: w35 -> [_ w884]
    tunnel: w31 -> [w555 _]
    tunnel: w29 -> [w511 _]
    tunnel: w28 -> [w500 _]
    tunnel: w27 -> [w508 _]
    tunnel: w26 -> [w512 _]
    tunnel: w25 -> [w510 _]
    tunnel: w24 -> [w506 _]
    tunnel: w14 -> [w504 _]
    tunnel: w13 -> [w503 _]
    tunnel: w1 -> [w502 _]
    frame False {
      # "aviのときだけ射影画像を出す。そうでないときは時間節約のため出さない"
      n253 = local read "folderpath"() -> (w505:path)
      n254 = local read "# of volumes"() -> (w498:dbl)
      n255 = case shown="\"avia.tif\"" w500 {
        tunnel: [w582 _ _ _] -> w554
        tunnel: [w581 _ _ _] -> w553
        tunnel: [_ w585 _ _] -> w550
        tunnel: [_ _ w592 _] -> w548
        tunnel: w505 -> [w575 w584 w588 _]
        tunnel: w502 -> [_ w583 _ _]
        frame "3DU16", Default {
          n256 = Strip Path(path=w575) -> (name=w578:string)  [unwired: 1 out]
          n257 = Concatenate Strings(w578, ".3DU16") -> (w576:string)
          n258 = Build Path(base path=w575, name or relative path=w576) -> (appended path=w579:path)
          n259 = Open/Create/Replace File(file path (use dialog)=w579, operation (0:open)=T11."replace or create") -> (refnum out=w581:refnum<file>, error out=w582:errorcluster)  [unwired: 4 in, 1 out]
        }
        frame "avi" {
          n260 = Build Path(base path=w584, name or relative path="3D-view.avi") -> (appended path=w587:path)
          n261 = call "IMAQ AVI2 Create"("Frames Per Second"=w583, "AVI Path"=w587) -> ("AVI Refnum"=w585:T16)  [unwired: 8 in, 1 out]
        }
        frame "avia.tif" {
          n262 = Strip Path(path=w588) -> (name=w590:string)  [unwired: 1 out]
          n263 = Concatenate Strings(w590, "aiviatif\\") -> (w589:string)
          n264 = Build Path(base path=w588, name or relative path=w589) -> (appended path=w595:path)
          n265 = call <vilib>:"Check if File or Folder Exists.vi"("path"=w595) -> ("error out"=w593:errorcluster, "file or folder exists?"=w594:bool, "dup path"=w592:path)  [unwired: 8 in]
          n266 = case shown="False" w594 {
            tunnel: w592 -> [w597 _]
            tunnel: w593 -> [w596 _]
            frame False {
              n267 = Create Folder(path (use dialog)=w597, error in=w596) -> ()  [unwired: 1 in, 3 out]
            }
            frame True {
            }
          }
        }
        frame "none" {
        }
      }
      n268 = Multiply(x=w511, y=w512) -> (x*y=w507:dbl)
      n269 = Compound Arithmetic op=ADD(w503, w510, w507) -> (w522:dbl)
      n270 = case shown="True" w513 {
        tunnel: [w557 w567] -> w517
        tunnel: w516 -> [w557 w565]
        tunnel: [w556 w566] -> w515
        tunnel: w514 -> [w556 w564]
        tunnel: w508 -> [_ w561]
        tunnel: w507 -> [_ w560]
        tunnel: w506 -> [_ w559]
        tunnel: w504 -> [_ w558]
        frame False {
        }
        frame True {
          n271 = Compound Arithmetic op=ADD(w558, w560, w559) -> (w563:dbl)
          n272 = Multiply(x=w563, y=w561) -> (x*y=w562:dbl)
          n273 = Set File Position(offset (in bytes) (0)=w562, refnum=w565, error in=w564) -> (refnum out=w567:refnum<file>, error out=w566:errorcluster)  [unwired: 1 in]
        }
      }
      n274 = Equal?(x=enum16{"3DU16", "avi", "avia.tif", "none"}."avi" ("save file 2"), y=w500) -> (x = y?=w499:bool)
      n275 = Subtract(x=w498, y=w511) -> (x-y=w539:dbl)
      n276 = Multiply(x=w522, y=w508) -> (x*y=w509:dbl)
      n277 = Select(t=w539, s="save all", f="# of vols to save") -> (s? t:f=w536:dbl)
      n278 = In Range and Coerce(upper limit=w498, x=w536, lower limit=0.0) -> (coerced(x)=w534:dbl)  [unwired: 1 out]
      n279 = Set File Position(offset (in bytes) (0)=w509, refnum=w521, error in=w519) -> (refnum out=w520:refnum<file>, error out=w518:errorcluster)  [unwired: 1 in]
      n280 = local read "z ofst"() -> (w540:dbl)
      n281 = for {
        N: w534 -> [w643]
        shift-right: [w655] -> w525
        shift-left: w518 -> [w657]
        shift-right: [w656] -> w526
        shift-left: w520 -> [w658]
        shift-right: [w620] -> w551
        shift-left: w554 -> [w654]
        shift-right: [w653] -> w552
        shift-left: w553 -> [w638]
        shift-right: [w650] -> w523
        shift-left: w517 -> [w652]
        shift-right: [w649] -> w524
        shift-left: w515 -> [w651]
        tunnel: w513 -> [w648]
        tunnel: w500 -> [w644]
        shift-right: [w636] -> w549
        shift-left: w550 -> [w637]
        tunnel: w548 -> [w634]
        tunnel: [w631] -> w547 mode=indexing
        tunnel: [w630] -> w546 mode=indexing
        tunnel: w555 -> [w598]
        tunnel: [w626] -> w545 mode=indexing
        shift-right: [w623] -> _
        shift-left: w540 -> [w624]
        tunnel: w511 -> [w622]
        shift-right: [w619] -> _
        shift-left: _ -> [w621]
        tunnel: [w603] -> w529 mode=concatenating
        tunnel: w499 -> [w600]
        i -> [w609]
        n282 = local read "auto z adjust"() -> (w628:T2)
        n283 = Bundle By Name(cluster=w628, "given ofst"=w624, "use given ofst"=TRUE) -> (w605:T2)
        n284 = Add(x=w622, y=w609) -> (x+y=w629:i64)
        "Numeric" <- w629
        n285 = flat-sequence {
          tunnel: w657 -> [w676]
          tunnel: w658 -> [w677]
          tunnel: [w677] -> w614
          tunnel: [w676] -> w613
          tunnel: [w675] -> w610
          tunnel: [w681] -> w617
          tunnel: [w680] -> w616
          tunnel: [w678] -> w615
          tunnel: w614 -> [w683]
          tunnel: w613 -> [w682]
          tunnel: [w692] -> w632
          tunnel: [w693] -> w655
          tunnel: [w694] -> w656
          tunnel: w617 -> [w694]
          tunnel: w616 -> [w693]
          tunnel: w615 -> [w692]
          tunnel: [w691] -> w611
          frame #0 {
            n286 = call <vilib>:"High Resolution Relative Seconds.vi"() -> ("relative seconds"=w675:dbl)
          }
          frame #1 {
            n287 = local read "frames per vol"() -> (w679:dbl)
            n288 = for {
              N: w679 -> [_]
              shift-right: [w690] -> w680
              shift-left: w682 -> [w689]
              shift-right: [w687] -> w681
              shift-left: w683 -> [w688]
              tunnel: [w685] -> w678 mode=indexing
              n289 = Read from Binary File(5:u16[][] [], 8:w689, 11:w688) -> (0:w690:errorcluster, 2:w686:u16[][], 3:w687:refnum<file>)  [unwired: 3 in, 1 out]
              n290 = call "reverse imageU16.vi"("output array in"=w686) -> ("output array out"=w685:u16[][])  [unwired: 2 in]
            }
          }
          frame #2 {
            n291 = call <vilib>:"High Resolution Relative Seconds.vi"() -> ("relative seconds"=w691:dbl)
          }
        }
        n292 = Subtract(x=w611, y=w610) -> (x-y=→"x-y 3":dbl)
        n293 = local read "coeffs"() -> (w601:bool)
        n294 = case shown="False" w601 {
          tunnel: w629 -> [_ w662]
          tunnel: [w659 w661] -> w602
          frame False {
            n295 = local read "static cropcalib ch1"() -> (w659:dbl[][][])
          }
          frame True {
            n296 = local read "img scan voltage"() -> (w666:dbl[][])
            n297 = local read "coeffs ch1"() -> (w665:T3)
            n298 = local read "man x correct"() -> (w663:dbl[])
            n299 = local read "mag correct"() -> (w660:dbl)
            n300 = local read "# of slices per frame"() -> (w664:dbl)
            n301 = local read "frames per vol"() -> (w668:dbl)
            n302 = local read "img scan tangent"() -> (w667:dbl[][])
            n303 = call "calc calib values from fitting (SubVI).vi"("mag correct"=w660, "# of slices"=w664, "man x correct"=w663, "# of pages"=w668, "volume index"=w662, "Cluster"=w665, "img scan voltage"=w666, "img scan tangent"=w667) -> ("Array"=w661:dbl[][][])  [unwired: 3 in]
          }
        }
        n304 = Equal To 0?(x=w609) -> (x = 0?=w640:bool)
        n305 = local read "correction"() -> (w599:T1)
        n306 = local read "cal"() -> (w633:bool)
        n307 = call "reconstruct 3D oblique image without config-2 (SubVI).vi"("correction"=w599, "auto z adjust"=w605, "image in"=w632, "config in"=w598, "cropcalib"=w633, "cropcalib data"=w602, "create 2D img"=w600) -> ("voxel number"=w642:i32[], "z ofst"=w625:dbl, "voxel size [um]"=w635:dbl[], "combined img"=w645:u16[][], "xyz"=w647:u16[][][])  [unwired: 1 in, 3 out]
        n308 = case shown="False" w648 {
          tunnel: w652 -> [_ w829]
          tunnel: w651 -> [_ w828]
          tunnel: [_ w827] -> w650
          tunnel: [_ w826] -> w649
          tunnel: w647 -> [w799 w824]
          tunnel: [w798 w823] -> w646
          tunnel: w645 -> [w797 w822]
          tunnel: [w796 w820] -> w639
          tunnel: w643 -> [w794 w819]
          tunnel: w642 -> [w793 w817]
          tunnel: [w790 w814] -> w641
          tunnel: w629 -> [_ w813]
          tunnel: [u16 0 w808] -> w630
          tunnel: w598 -> [_ w807]
          tunnel: w605 -> [_ w806]
          tunnel: w602 -> [w788 w805]
          tunnel: [w787 w804] -> w604
          tunnel: w600 -> [_ w801]
          frame False {
            n309 = Build Array(w794, 1) -> (w791:i32[])
            n310 = Build Array(w797) -> (w796:u16[][][])
            n311 = Build Array(w799) -> (w798:u16[][][][])
            n312 = Insert Into Array(array=w793, index=0, new element=w791) -> (w790:i32[])
            n313 = Build Array(w788) -> (w787:dbl[][][][])
          }
          frame True {
            n314 = local read "frames per vol"() -> (w830:dbl)
            n315 = for {
              N: w830 -> [_]
              shift-right: [w845] -> w826
              shift-left: w828 -> [w846]
              shift-right: [w844] -> w827
              shift-left: w829 -> [w847]
              tunnel: [w842] -> w809 mode=indexing
              n316 = Read from Binary File(5:u16[][] [], 8:w846, 11:w847) -> (0:w845:errorcluster, 2:w843:u16[][], 3:w844:refnum<file>)  [unwired: 3 in, 1 out]
              n317 = local read "h shift"() -> (w850:i32)
              n318 = local read "v shift"() -> (w849:i32)
              n319 = call "reverse imageU16.vi"("output array in"=w843, "reverse h"=TRUE ("reverse h 2")) -> ("output array out"=w851:u16[][])  [unwired: 1 in]
              n320 = call "image shift (SubVI).vi"("v shift"=w849, "h shift"=w850, "Array in"=w851) -> ("Array out"=w842:u16[][])  [unwired: 8 in]
            }
            n321 = Build Array(w819, 2) -> (w815:i32[])
            n322 = local read "coeffs"() -> (w802:bool)
            n323 = case shown="False" w802 {
              tunnel: w813 -> [_ w835]
              tunnel: [w831 w833] -> w803
              frame False {
                n324 = local read "static cropcalib ch2"() -> (w831:dbl[][][])
              }
              frame True {
                n325 = local read "img scan voltage"() -> (w838:dbl[][])
                n326 = local read "coeffs ch2"() -> (w839:T3)
                n327 = local read "mag corr ch2"() -> (w832:dbl)
                n328 = local read "# of slices per frame"() -> (w840:dbl)
                n329 = local read "frames per vol"() -> (w836:dbl)
                n330 = local read "img scan tangent"() -> (w837:dbl[][])
                n331 = local read "man x correct"() -> (w834:dbl[])
                n332 = call "calc calib values from fitting (SubVI).vi"("mag correct"=w832, "# of slices"=w840, "man x correct"=w834, "# of pages"=w836, "volume index"=w835, "Cluster"=w839, "img scan voltage"=w838, "img scan tangent"=w837) -> ("Array"=w833:dbl[][][])  [unwired: 3 in]
              }
            }
            n333 = local read "y shift comp ch2"() -> (w811:dbl)
            n334 = Bundle By Name(cluster=w807, "3D reconst config.y shift comp"=w811) -> (w810:T4)
            n335 = local read "correction"() -> (w800:T1)
            n336 = local read "cal"() -> (w812:bool)
            n337 = call "reconstruct 3D oblique image without config-2 (SubVI).vi"("correction"=w800, "auto z adjust"=w806, "image in"=w809, "config in"=w810, "cropcalib"=w812, "cropcalib data"=w803, "create 2D img"=w801) -> ("combined img"=w821:u16[][], "xyz"=w825:u16[][][])  [unwired: 1 in, 6 out]
            n338 = Build Array(w822, w821) -> (w820:u16[][][])
            n339 = Build Array(w805, w803) -> (w804:dbl[][][][])
            n340 = Build Array(w824, w825) -> (w823:u16[][][][])
            n341 = Array Max & Min(array=w809) -> (max value=w808:u16)  [unwired: 3 out]
            n342 = Insert Into Array(array=w817, index=0, new element=w815) -> (w814:i32[])
          }
        }
        n343 = case shown="\"3DU16\", Default" w644 {
          tunnel: w654 -> [w709 w739 w777 _]
          tunnel: [w713 w736 w776 _] -> w620
          tunnel: [w712 _ _ _] -> w653
          tunnel: w646 -> [w711 _ w780 _]
          tunnel: w635 -> [w707 _ _ _]
          tunnel: w641 -> [w706 _ _ _]
          tunnel: w640 -> [w705 _ w757 _]
          tunnel: w639 -> [_ w742 _ _]
          tunnel: w638 -> [w704 _ _ _]
          tunnel: w637 -> [_ w738 _ _]
          tunnel: [_ w737 _ _] -> w636
          tunnel: w629 -> [_ _ w773 _]
          tunnel: w634 -> [_ _ w761 _]
          tunnel: w598 -> [_ _ w770 _]
          frame "3DU16", Default {
            n344 = case shown="False" w705 {
              tunnel: [w726 w734] -> w710
              tunnel: w709 -> [w727 w733]
              tunnel: [w727 w731] -> w708
              tunnel: w707 -> [_ w730]
              tunnel: w706 -> [_ w729]
              tunnel: w704 -> [w726 w728]
              frame False {
              }
              frame True {
                n345 = Write to Binary File(file (use dialog)=w728, data=w730, error in=w733) -> (refnum out=w735:refnum<file>, error out=w732:errorcluster)  [unwired: 3 in, 1 out]
                n346 = Write to Binary File(file (use dialog)=w735, data=w729, error in=w732) -> (refnum out=w734:refnum<file>, error out=w731:errorcluster)  [unwired: 3 in, 1 out]
              }
            }
            n347 = flat-sequence {
              tunnel: w708 -> [w715]
              tunnel: w710 -> [w716]
              tunnel: w711 -> [w717]
              tunnel: [w717] -> w701
              tunnel: [w716] -> w700
              tunnel: [w715] -> w699
              tunnel: [w714] -> w698
              tunnel: [w722] -> w703
              tunnel: [w721] -> w702
              tunnel: w701 -> [w720]
              tunnel: w700 -> [w719]
              tunnel: w699 -> [w718]
              tunnel: [w724] -> w712
              tunnel: [w725] -> w713
              tunnel: w703 -> [w725]
              tunnel: w702 -> [w724]
              tunnel: [w723] -> w697
              frame #0 {
                n348 = call <vilib>:"High Resolution Relative Seconds.vi"() -> ("relative seconds"=w714:dbl)
              }
              frame #1 {
                n349 = Write to Binary File(file (use dialog)=w719, data=w720, error in=w718) -> (refnum out=w721:refnum<file>, error out=w722:errorcluster)  [unwired: 3 in, 1 out]
              }
              frame #2 {
                n350 = call <vilib>:"High Resolution Relative Seconds.vi"() -> ("relative seconds"=w723:dbl)
              }
            }
            n351 = Subtract(x=w697, y=w698) -> (x-y=→"x-y":dbl)
          }
          frame "avi" {
            w740 = T17 4 items=["Grayscale (U8)", "Grayscale (I16)", "Grayscale (SGL)", "Complex (CSG)", "RGB (U32)", "HSL (U32)", "RGB (U64)", "Grayscale (U16)"] ("Image Type")
            n352 = local read "Cluster 2"() -> (w748:T5)
            n353 = call "IMAQ Create"("Image Name"="xx", "Image Type"=w740) -> ("New Image"=w747:T18, "error out"=w745:errorcluster)  [unwired: 3 in]
            n354 = Unbundle(w748) -> ("colors 2"=w749:T19, "on/off 2"=w751:bool[], "fast/slow"=w750:bool)  [unwired: 1 out]
            n355 = call "multicolor creation 3(subvi).vi"("on/off"=w751, "colors"=w749, "fast/slow"=w750, "img array in"=w742) -> ("mixed img array"=w752:u32[][])  [unwired: 4 in, 1 out]
            n356 = call "IMAQ ArrayToColorImage"("Image Pixels (U32)"=w752, "Image"=w747, "error in (no error)"=w745) -> ("Image Out"=w744:T18, "error out"=w746:errorcluster)  [unwired: 2 in]
            n357 = call "IMAQ AVI2 Write Frame"("error in (no error)"=w739, "Image"=w744, "AVI Refnum"=w738) -> ("error out"=w736:errorcluster, "Image Out (duplicate)"=w743:T18, "AVI Refnum (duplicate)"=w737:T16)  [unwired: 6 in]
            n358 = call "IMAQ Dispose"("Image"=w743, "error in (no error)"=w746) -> ()  [unwired: 4 in, 1 out]
          }
          frame "avia.tif" {
            n359 = local read "folderpath"() -> (w771:path)
            n360 = Unbundle By Name(w770) -> ("3D reconst config.xy cut ofst"=w764:dbl, "3D reconst config.voxel size xy[um]"=w762:dbl, "3D reconst config.oblique angle [deg]"=w768:dbl)
            n361 = Number To Decimal String(number=w773) -> (decimal integer string=w772:string)  [unwired: 1 in]
            n362 = Strip Path(path=w771) -> (name=w778:string)  [unwired: 1 out]
            n363 = Concatenate Strings(w778, "_t" ("string"), w772, ".aivia.tif") -> (w779:string)
            n364 = Build Path(base path=w761, name or relative path=w779) -> (appended path=w756:path)
            n365 = Compound Arithmetic op=MULTIPLY(w768, invert 180.0, 3.141592653589793) -> (w766:dbl)
            n366 = Sine(x=w766) -> (sin(x)=w765:dbl)
            n367 = call <vilib>:"Check if File or Folder Exists.vi"("path"=w756) -> ("file or folder exists?"=w754:bool, "dup path"=w755:path)  [unwired: 8 in, 1 out]
            n368 = case shown="False" w754 {
              tunnel: w755 -> [w781 w783]
              tunnel: [w781 w782] -> w753
              frame False {
              }
              frame True {
                n369 = Delete(path (use dialog)=w783) -> (deleted path=w782:path)  [unwired: 4 in, 2 out]
              }
            }
            n370 = Compound Arithmetic op=MULTIPLY(w764, w762, w765) -> (w763:dbl)
            n371 = Build Array(w763, w762) -> (w758:dbl[])
            n372 = Build Path(base path=w761, name or relative path="zofst.csv") -> (appended path=w759:path)
            n373 = call "write aviatif file (SubVI).vi"("error in"=w777, "img data"=w780, "path"=w753) -> ("error out"=w776:errorcluster)  [unwired: 8 in]
            n374 = case shown="True" w757 {
              tunnel: w759 -> [_ w786]
              tunnel: w758 -> [_ w785]
              frame False {
              }
              frame True {
                n375 = call-poly <vilib>:"Write Delimited Spreadsheet.vi"("file path (dialog if empty)"=w786, "format (%.3f)"="%.6f", "1D data"=w785) -> ()  [unwired: 11 in, 2 out]
              }
            }
          }
          frame "none" {
          }
        }
        n376 = Quotient & Remainder(x=w609, y=10) -> (x-y*floor(x/y)=w607:i32)  [unwired: 1 out]
        n377 = Equal To 0?(x=w607) -> (x = 0?=w606:bool)
        n378 = case shown="False" w606 {
          tunnel: w625 -> [_ w674]
          tunnel: w624 -> [w669 w673]
          tunnel: [w669 w670] -> w623
          frame False {
          }
          frame True {
            n379 = Decrement(x=w673) -> (x-1=w671:dbl)
            n380 = Increment(x=w673) -> (x+1=w672:dbl)
            n381 = In Range and Coerce(upper limit=w672, x=w674, lower limit=w671) -> (coerced(x)=w670:dbl)  [unwired: 1 out]
          }
        }
        n382 = call "create coeffs(subVI).vi"("auto z adjust"=w605, "Array in"=w604, "config in"=w598) -> ("Array out"=w603:dbl[][])  [unwired: 8 in]
        n383 = To Unsigned Word Integer(number=w623) -> (unsigned 16bit integer=w626:u16)
        n384 = flat-sequence {
          tunnel: [w695] -> w619
          tunnel: w620 -> [_]
          frame #0 {
            n385 = call <vilib>:"High Resolution Relative Seconds.vi"() -> ("relative seconds"=w695:dbl)
          }
        }
        n386 = Subtract(x=w619, y=w621) -> (x-y=→"x-y 2":dbl)
        n387 = Array Max & Min(array=w632) -> (max value=w631:u16)  [unwired: 3 out]
      }
      "Array" <- w547
      "Array 2" <- w546
      "Waveform Graph 8" <- w547
      "Waveform Graph 7" <- w546
      "Waveform Graph 3" <- w545
      n388 = Close File(refnum=w526, error in=w525) -> ()  [unwired: 2 out]
      n389 = case shown="True" w513 {
        tunnel: w524 -> [_ w569]
        tunnel: w523 -> [_ w568]
        frame False {
        }
        frame True {
          n390 = Close File(refnum=w568, error in=w569) -> ()  [unwired: 2 out]
        }
      }
      n391 = case shown="\"avia.tif\"" w500 {
        tunnel: w552 -> [w572 _ _ _]
        tunnel: w551 -> [w571 w573 _ _]
        tunnel: w549 -> [_ w574 _ _]
        tunnel: [w570 _ _ _] -> w533
        frame "3DU16", Default {
          n392 = Close File(refnum=w572, error in=w571) -> (path=w570:path)  [unwired: 1 out]
        }
        frame "avi" {
          n393 = call "IMAQ AVI2 Close"("error in (no error)"=w573, "AVI Refnum"=w574) -> ()  [unwired: 9 in, 1 out]
        }
        frame "avia.tif" {
        }
        frame "none" {
        }
      }
      "path" <- w533
      n394 = local read "folderpath"() -> (w530:path)
      n395 = Build Array(w547, w546, w545) -> (w541:u16[][])
      n396 = local read "folderpath"() -> (w544:path)
      n397 = Build Path(base path=w530, name or relative path="cropparameters.csv") -> (appended path=w532:path)
      n398 = call-poly <vilib>:"Write Delimited Spreadsheet.vi"("file path (dialog if empty)"=w532, "format (%.3f)"="%.6f", "2D data"=w529, "delimiter (\\t)"="," ("delimiter (\\t)")) -> ()  [unwired: 10 in, 2 out]
      n399 = Build Path(base path=w544, name or relative path="profile(ch0ch1intensity and z adj)-2.csv") -> (appended path=w542:path)
      n400 = call-poly <vilib>:"Write Delimited Spreadsheet.vi"("file path (dialog if empty)"=w542, "2D data"=w541) -> ()  [unwired: 12 in, 2 out]
    }
    frame True {
      w905 = "-cropbulkcalib" ("regular expression")
      # "imgcalib.txtファイルを生成"
      # "crop calibration用データホルダ名の末尾に-cropcalibをつける。すでにある場合はしない。"
      n401 = case shown="False" w894 {
        selector: w894 -> [w937 w940]
        tunnel: [w937 w940] -> w893
        frame False {
          n402 = One Button Dialog(message="Delete calib files and try again.") -> (true=w938:bool)  [unwired: 1 in]
          n403 = Stop(stop? (T)=w938) -> ()
        }
        frame True {
        }
      }
      n404 = for {
        N: w884 -> [_]
        tunnel: [w951] -> w920 mode=indexing
        tunnel: w888 -> [w966]
        shift-right: [w963] -> w902
        shift-left: w901 -> [w959]
        shift-right: [w964] -> w903
        shift-left: w900 -> [w957]
        tunnel: w885 -> [w948]
        shift-right: [w942] -> _
        shift-left: dbl[][][] [] ("optimized parameters") -> [w950]
        tunnel: w886 -> [w945]
        tunnel: [w944] -> w897 mode=indexing
        tunnel: w896 -> [w943]
        tunnel: w893 -> [_]
        i -> [w947]
        n405 = Multiply(x=w948, y=w947) -> (x*y=w946:i32)
        n406 = local read "int frame ch1"() -> (w953:dbl)
        n407 = local read "bytes per frame"() -> (w961:i64)
        n408 = local read "frames per vol"() -> (w955:dbl)
        n409 = Add(x=w945, y=w946) -> (x+y=w944:i32)
        n410 = Not Equal To 0?(x=w947) -> (x != 0?=w949:bool)
        n411 = Compound Arithmetic op=MULTIPLY(w944, w955) -> (w954:dbl)
        n412 = Add(x=w953, y=w954) -> (x+y=w952:dbl)
        n413 = Multiply(x=w952, y=w961) -> (x*y=w960:dbl)
        n414 = local read "frames per vol"() -> (w965:dbl)
        n415 = Set File Position(offset (in bytes) (0)=w960, refnum=w957, error in=w959) -> (refnum out=w956:refnum<file>, error out=w958:errorcluster)  [unwired: 1 in]
        n416 = for {
          N: w965 -> [_]
          tunnel: [w968] -> w962 mode=indexing
          shift-right: [w973] -> w963
          shift-left: w958 -> [w975]
          shift-right: [w972] -> w964
          shift-left: w956 -> [w974]
          n417 = Read from Binary File(5:u16[][] [], 8:w975, 11:w974) -> (0:w973:errorcluster, 2:w970:u16[][], 3:w972:refnum<file>)  [unwired: 3 in, 1 out]
          n418 = call "reverse imageU16.vi"("output array in"=w970) -> ("output array out"=w969:u16[][])  [unwired: 2 in]
          n419 = local read "mag correct"() -> (w967:dbl)
          n420 = call "horizontal mag adjust.vi"("2D mag correct"=w967, "Array in"=w969) -> ("Array out"=w968:u16[][])  [unwired: 9 in]
        }
        n421 = call "optimize crop parameters-3 (SubVI).vi"("ref image in"=w943, "fit results"="fit results", "init values"=w950, "use external int values"=w949, "config in"=w966, "image in"=w962) -> ("opt param for feedback"=w942:dbl[][][], "optimized parameters"=w951:dbl[][][])  [unwired: 4 in]
        "calib index" <- w947
      }
      n422 = case shown="True" w921 {
        tunnel: w922 -> [_ w992]
        tunnel: w899 -> [_ w993]
        tunnel: w888 -> [_ w999]
        tunnel: w920 -> [w986 w998]
        tunnel: [w985 w996] -> w869
        tunnel: w885 -> [_ w991]
        tunnel: w884 -> [_ w990]
        tunnel: w886 -> [_ w989]
        tunnel: w895 -> [_ w987]
        frame False {
          n423 = Build Array(w986) -> (w985:dbl[][][][][])
        }
        frame True {
          n424 = for {
            N: w990 -> [_]
            tunnel: w999 -> [w1026]
            tunnel: [w1011] -> w997 mode=indexing
            shift-right: [w1023] -> w994
            shift-left: w993 -> [w1021]
            shift-right: [w1024] -> w995
            shift-left: w992 -> [w1020]
            tunnel: w991 -> [w1006]
            shift-right: [w1002] -> _
            shift-left: dbl[][][] [] ("optimized parameters") -> [w1010]
            tunnel: w989 -> [w1005]
            tunnel: w987 -> [w1003]
            i -> [w1007]
            n425 = local read "bytes per frame"() -> (w1014:i64)
            n426 = local read "frames per vol"() -> (w1015:dbl)
            n427 = local read "int frame ch2"() -> (w1013:dbl)
            n428 = Multiply(x=w1006, y=w1007) -> (x*y=w1008:i32)
            n429 = Add(x=w1005, y=w1008) -> (x+y=w1004:i32)
            n430 = Not Equal To 0?(x=w1007) -> (x != 0?=w1009:bool)
            n431 = Compound Arithmetic op=MULTIPLY(w1004, w1015) -> (w1016:dbl)
            n432 = Add(x=w1013, y=w1016) -> (x+y=w1017:dbl)
            n433 = local read "frames per vol"() -> (w1025:dbl)
            n434 = Multiply(x=w1017, y=w1014) -> (x*y=w1012:dbl)
            n435 = Set File Position(offset (in bytes) (0)=w1012, refnum=w1020, error in=w1021) -> (refnum out=w1019:refnum<file>, error out=w1018:errorcluster)  [unwired: 1 in]
            n436 = for {
              N: w1025 -> [_]
              tunnel: [w1034] -> w1022 mode=indexing
              shift-right: [w1037] -> w1023
              shift-left: w1018 -> [w1039]
              shift-right: [w1036] -> w1024
              shift-left: w1019 -> [w1038]
              n437 = Read from Binary File(5:u16[][] [], 8:w1039, 11:w1038) -> (0:w1037:errorcluster, 2:w1033:u16[][], 3:w1036:refnum<file>)  [unwired: 3 in, 1 out]
              n438 = local read "h shift"() -> (w1029:i32)
              n439 = local read "v shift"() -> (w1028:i32)
              n440 = call "reverse imageU16.vi"("output array in"=w1033, "reverse h"=TRUE ("reverse h 2")) -> ("output array out"=w1032:u16[][])  [unwired: 1 in]
              n441 = local read "mag corr ch2"() -> (w1027:dbl)
              n442 = call "image shift (SubVI).vi"("v shift"=w1028, "h shift"=w1029, "Array in"=w1032) -> ("Array out"=w1035:u16[][])  [unwired: 8 in]
              n443 = call "horizontal mag adjust.vi"("2D mag correct"=w1027, "Array in"=w1035) -> ("Array out"=w1034:u16[][])  [unwired: 9 in]
            }
            n444 = local read "fit results"() -> (w1001:bool)
            n445 = call "optimize crop parameters-3 (SubVI).vi"("ref image in"=w1003, "fit results"=w1001, "init values"=w1010, "use external int values"=w1009, "config in"=w1026, "image in"=w1022) -> ("opt param for feedback"=w1002:dbl[][][], "optimized parameters"=w1011:dbl[][][])  [unwired: 4 in]
          }
          n446 = Close File(refnum=w995, error in=w994) -> (error out=w1000:errorcluster)  [unwired: 1 out]
          n447 = call <vilib>:"Simple Error Handler.vi"("error in (no error)"=w1000) -> ()  [unwired: 4 in, 5 out]
          n448 = Build Array(w998, w997) -> (w996:dbl[][][][][])
        }
      }
      n449 = Close File(refnum=w903, error in=w902) -> (error out=w923:errorcluster)  [unwired: 1 out]
      n450 = call <vilib>:"Simple Error Handler.vi"("error in (no error)"=w923) -> ("error out"=w904:errorcluster)  [unwired: 4 in, 4 out]
      n451 = Array Size(array=w869) -> (size(s)=w883:i32[])
      n452 = Unbundle By Name(w888) -> ("AOD scan speed ratio"=w867:dbl)
      n453 = Index Array(array=w883) -> (element #3=w870:i32, element #4=w871:i32)  [unwired: 4 in, 2 out]
      n454 = Build Path(base path=w887, name or relative path="cropbulkcalib.cal") -> (appended path=w911:path)
      n455 = Bundle By Name(cluster=T9 {"config cluster"={"xy cut pos correct"=[], "3D reconst config"={"xyz pos"=[], "color 4"={"color array"=[], "num of colors"=0, "max"=0.0, "min"=0.0}, "autogain"=FALSE, "zoom"=0.0, "slice(T)/stack(F)"=FALSE, "xy cut mag"=0.0, "xy cut ofst"=0.0, "z/xy comp"=0.0, "y shift comp"=0.0, "max plot"=FALSE, "oblique angle [deg]"=0.0, "voxel size z [um]"=0.0, "voxel size xy[um]"=0.0, "reverse v"=FALSE, "reverse h"=FALSE, "3D reconstruction"=FALSE, "reverse z"=FALSE}, "xy cut pos"=[], "AOD scan speed ratio"=0.0, "Nx"=0.0, "stack method"=enum."0pad to z", "y shift"=0}, "optimized param"=[], "volume indices"=[]}, "config cluster"=w888, "optimized param"=w869, "volume indices"=w897) -> (w915:T9)
      n456 = for {
        tunnel: w870 -> [w927]
        tunnel: w871 -> [w926]
        tunnel: [w925] -> w872 mode=concatenating
        tunnel: w869 -> [w924] mode=indexing
        n457 = for {
          N: w926 -> [_]
          tunnel: w924 -> [w931]
          tunnel: [w929] -> w925 mode=concatenating
          tunnel: w927 -> [w928]
          i -> [w930]
          n458 = for {
            N: w928 -> [_]
            tunnel: w931 -> [w936]
            tunnel: w930 -> [w934]
            tunnel: [w935] -> w929 mode=indexing
            i -> [w933]
            n459 = Index Array(array=w936, index (dim 0)=0 ("disabled index (vol)"), index (dim 1)=w933, index (dim 2)=w934) -> (element=w935:dbl[])  [unwired: 1 in]
          }
        }
      }
      n460 = Open/Create/Replace File(file path (use dialog)=w911, error in=w904, operation (0:open)=T11."replace or create") -> (refnum out=w918:refnum<file>, error out=w919:errorcluster)  [unwired: 3 in, 1 out]
      n461 = Write to Binary File(file (use dialog)=w918, data=w915, error in=w919) -> (refnum out=w917:refnum<file>, error out=w916:errorcluster)  [unwired: 3 in, 1 out]
      n462 = Index Array(array=w872, index (col) #1=0 ("disabled index (col)"), index (col) #2=1 ("index (col)"), index (col) #3=2 ("index (col)"), index (col) #4=3 ("index (col)")) -> (element #1=w881:dbl[], element #2=w876:dbl[], element #4=w875:dbl[])  [unwired: 4 in, 1 out]
      n463 = Add(x=w867, y=w881) -> (x+y=w877:dbl[])
      n464 = Close File(refnum=w917, error in=w916) -> (error out=w909:errorcluster)  [unwired: 1 out]
      n465 = Build Array(w877, w876, dbl[] [] ("element"), w875) -> (w874:dbl[][])
      n466 = Transpose 2D Array(2D array=w874) -> (transposed array=w868:dbl[][])
      n467 = Build Path(base path=w887, name or relative path="cropcalib.csv") -> (appended path=w891:path)
      n468 = call-poly <vilib>:"Write Delimited Spreadsheet.vi"("file path (dialog if empty)"=w891, "format (%.3f)"="%.6f", "2D data"=w868, "delimiter (\\t)"="," ("delimiter (\\t)")) -> ("error out"=w853:errorcluster)  [unwired: 10 in, 1 out]
      n469 = local read "3D config"() -> (w866:T7)
      n470 = Unbundle By Name(w866) -> ("voxel size xy[um]"=w865:dbl, "voxel size z [um]"=w864:dbl, "y shift comp"=w863:dbl)
      n471 = local read "y shift comp ch2"() -> (w862:dbl)
      n472 = local read "folderpath"() -> (w858:path)
      n473 = local read "h shift"() -> (w861:i32)
      n474 = local read "v shift"() -> (w860:i32)
      n475 = Strip Path(path=w887) -> (stripped path=w910:path, name=w907:string)
      n476 = Build Array(w865, w864, w863, w862, w861, w860) -> (w859:dbl[])
      n477 = Build Path(base path=w858, name or relative path="imgcalib.txt") -> (appended path=w857:path)
      n478 = Match Pattern(string=w907, regular expression=w905) -> (match substring=w908:string)  [unwired: 1 in, 3 out]
      n479 = call-poly <vilib>:"Write Delimited Spreadsheet.vi"("file path (dialog if empty)"=w857, "format (%.3f)"="%.6f", "1D data"=w859, "error in (no error)"=w853, "delimiter (\\t)"="\r\n") -> ("error out"=w852:errorcluster)  [unwired: 9 in, 1 out]
      n480 = Not Equal?(x=w908, y=w905) -> (x != y?=w906:bool)
      n481 = case shown="True" w906 {
        tunnel: w910 -> [_ w984]
        tunnel: w887 -> [_ w978]
        tunnel: w909 -> [_ w981]
        tunnel: w907 -> [_ w980]
        tunnel: w905 -> [_ w979]
        tunnel: w852 -> [_ _]
        frame False {
        }
        frame True {
          n482 = Concatenate Strings(w980, w979) -> (w983:string)
          n483 = local write "first calib?"(FALSE ("first calib?")) -> ()
          n484 = Build Path(base path=w984, name or relative path=w983) -> (appended path=w976:path)
          n485 = Move(source path=w978, error in=w981, 10:w976) -> (error out=→"error out":errorcluster)  [unwired: 2 in, 2 out]
          n486 = local write "folderpath"(w976) -> ()
          n487 = local write "calib folder"(w976) -> ()
        }
      }
    }
  }
